vi "190717-FileSheduledROBOTPres-Ardu-TREATchoice_Prince_ArduinoWait.vi"() -> ()   [LabVIEW 2016]
uses:
  <vilib>/sound2/lvsound2.llb/Sampling Mode.ctl
  <vilib>/sound2/lvsound2.llb/Sound Data Format.ctl
  <vilib>/Utility/file.llb/Read From Spreadsheet File (string).vi
  <vilib>/Instr/_visa.llb/VISA Configure Serial Port (Instr).vi
  <vilib>/Utility/file.llb/Read From Spreadsheet File (DBL).vi
  <vilib>/sound2/lvsound2.llb/Sound Output Write (DBL).vi
panel:
  out "Numeric Control 2":i32
  out "number":i32=1
  in  "file path (dialog if empty)":path=path "C:/Users/Ralph/Documents/roboNew/RobotFiles/new files/787/RoboTutoringSchedule787.csv"
  in  "filename":string="787_undir_1766_3527_song1"
  out "all rows":string[][](array[string])=[["15:24", "787_undir_1766_3527_call1", "2", "a"], ["15:15", "787_undir_1766_3527_headmovement1", "1", "v"], ["15:16", "787_undir_1766_3527_song1", "2", "v"], ["15:17", "787_undir_1766_3527_song2", "2", "av"], ["15:18", "787_undir_1766_3527headmovement2", "3", "av"], ["15:19", "787_undir_1766_3527_call1", "4", "v"], ["15:20", "787_undir_1766_3527_song2", "2", "a"]]
  in  "Stop Button1":bool
  in  "Timer active":bool=TRUE
  in  "testPlay":bool
  in  "stop 2":bool
  out "signal":waveform(dbl)[](graph)=[{"t0"=timestamp(0 s since 1904-01-01), "dt"=0.008333333333333333, "Y"=array[729 elements]}, {"t0"=timestamp(0 s since 1904-01-01), "dt"=0.008333333333333333, "Y"=array[729 elements]}, {"t0"=timestamp(0 s since 1904-01-01), "dt"=2.0833333333333333e-05, "Y"=array[292292 elements]}, {"t0"=timestamp(0 s since 1904-01-01), "dt"=2.0833333333333333e-05, "Y"=array[292292 elements]}]
  out "Numeric 3":i32
  in  "sheduled from list":bool
  in  "play (sec)":dbl format="%#_13g"
  in  "play for (min)":dbl=30.0 format="%#_13g"
  in  "Absolute Date Time":bool=TRUE
  in  "play until":timestamp=timestamp(3577784880.043 s since 1904-01-01)
  in  "Tab Control":T1(tab)=enum."calibrations"
  in  "pause in between 1 and (sec)":dbl=6.0 format="%#_13g"
  out "Zufallszahl":dbl=1.0
  out "Numeric Control":i32=14
  in  "y":dbl=3.5
  in  "y 2":dbl=7.0
  in  "random pause":bool
  in  "constant pause":dbl=1.0
  in  "VISA resource name":refnum<visa-resource-name>="COM5"
  out "path":path=path "C:/Users/Ralph/Documents/roboNew/RobotFiles/new files/787/wav/787_undir_1766_3527_song1.wav"
  in  "excelListoutput 2":string[](array[string])
  out "Time at End":timestamp=timestamp(3646218925.390868 s since 1904-01-01)
  in  "protocol-file":path=path "C:/Users/Ralph/Documents/RobotFiles/robot1/protokol/robo1.txt"
  out "EOF? 2":bool
  in  "txt path":path=path "C:/Users/Ralph/Documents/roboNew/RobotFiles/new files/787/txt"
  in  "wav path":path=path "C:/Users/Ralph/Documents/roboNew/RobotFiles/new files/787/wav"
  in  "play clips in random order":bool=TRUE
  in  "Operation (0:Öffnen)":T2(ring)=enum."open or create"
  out "file in use 2":path=path "C:/Users/Ralph/Documents/roboNew/RobotFiles/new files/787/txt/787_undir_1766_3527_song1.txt"
  out "excelListoutput":string[](array[string])
  out "filenames":string[](array[string])=["._787_undir_1766_3527_call1.txt", "._787_undir_1766_3527_headmovement1.txt", "._787_undir_1766_3527_song1.txt", "._787_undir_1766_3527_song2.txt", "._787_undir_1766_3527headmovement2.txt", "._787_undir_1771_3532_call2.txt", "787_undir_1766_3527_call1.txt", "787_undir_1766_3527_headmovement1.txt", "787_undir_1766_3527_headmovement2.txt", "787_undir_1766_3527_song1.txt", "787_undir_1766_3527_song2.txt", "787_undir_1766_3527_song3.txt", "787_undir_1766_3527headmovement2.txt", "787_undir_1771_3532_call2.txt"]
  out "Fehler (Ausgang)":errorcluster
  out "element":i32=729
  out "size(s) 2":i32[](array[numeric])=[729, 4]
  out "Zufallszahl 2":dbl
  in  "00:00":string[](array[string])=["00:00", "902_3218_song1", "2", "2,5", "3"]
  in  "#songs if stop or manual":i32=1
  in  "delay in frames default":i32
  in  "delay in intro":i32=20
  in  "delay in frames contact":i32=35
  in  "delay in head":i32
  in  "delay in frames song":i32=19
  out "substring":string="787_un"
  in  "AttenBeak":dbl(slide)=0.5868263473053893 scale=0.0..2.0
  in  "OffsetB":dbl(slide)=4.407185628742515 scale=-2.0..8.0
  in  "AttenuateH":dbl(slide)=0.3413173652694611 scale=0.0..1.0
  in  "OffsetH":dbl(slide)=15.62874251497006 scale=0.0..30.0
  in  "Endwert Motor beak":dbl=3.0
  in  "Sampling Rate Hz":i32=120
  in  "negateBeak":bool
  in  "arduino first":bool
  in  "Endwert Motor Head":dbl
  in  "negateHead":bool=TRUE
  in  "delay movemet (samples'":dbl
  in  "wait after arduino":u32=1
  in  "wait before arduino":u32=1000
  out "error out":errorcluster
  out "error out 2":errorcluster
  out "head":dbl[](graph)=[3.25524556, 3.25294984, 3.251120901, 3.253046538, 3.254022268, 3.249303827, 3.249215039, 3.2499700590000002, 3.2493095459999997, 3.248565229, 3.2495452080000002, 3.2534044619999998, 3.256207934, 3.259231787, 3.2619914740000002, 3.264856742, 3.270676864, 3.2746376670000004, 3.284129863, 3.2956746199999998, 3.300381861, 3.312177085, 3.321709216, 3.3253852939999997, 3.327262519, 3.3293910859999998, 3.331196512, 3.331579734, 3.330605733, 3.334049257, 3.333645644, 3.334527532, 3.336280094, 3.338991439, 3.3986287020000003, 3.708982361, 4.4244339859999995, 5.395669363, 4.981378934, 5.531567489, 5.848262042, 6.068882211, 6.201616043, 6.242202127, 6.294738485, 6.294786435, 6.306837376000001, 6.284361685, 6.263991517, 6.244760256, 6.225402722, 6.220988522, 6.193365955, 6.197575853, 6.179223407, 6.186652073, 6.186890815, 6.173817251, 6.173178823, 6.175700391, 6.164617732, 6.166750807, 6.167856604, 6.167219086, 6.1790438850000005, 6.184330803, 6.183288790000001, 6.182242962, 6.199099487, 6.195969857000001, 6.201212773, 6.184360826000001, 6.194674002999999, 6.1892039510000005, 6.199708998, 6.190704289, 6.189952258, 6.18540825, 6.1763629689999995, 6.172376483000001, 6.150909639, 6.150504311, 6.14149011, 6.149450419, 6.139135842, 6.132062482, 6.132533071, 6.109822698, 6.114936618, 6.0545361589999995, 5.783199583, 6.732510575, 5.991935586, 5.328017849, 4.880723553999999, 4.649590938999999, 4.510889999, 4.42124256, 4.36307795, 4.3398573119999995, 4.3296939000000005, 4.326524216, 4.336089037, 4.352689383, 4.363369283, 4.367219745, 4.372433282, 4.384251809, 4.366195183, 4.371260579, 4.414009236, 4.412001181, 4.382009835, 4.405984394, 4.381107668, 4.3987839840000005, 4.39187896, 4.392596929, 4.387452412, 4.40148303, 4.407740435, 4.419200268, 4.418066569, 4.395799583, 4.414641294, 4.425368311, 4.4292789169999995, 4.424837557, 4.436759943, 4.427485776, 4.417763665, 4.42740788, 4.434259032, 4.443666318, 4.440932629, 4.438029218, 4.430423928, 4.437210477, 4.42934142, 4.4440042150000005, 4.46085612, 4.515481544, 4.599755559, 4.7746048, 5.147768213, 5.608406523999999, 5.970478003, 6.283057851, 6.451734065, 6.544220087999999, 6.597438406999999, 6.604634316, 6.6057426889999995, 6.607558951, 6.603214268, 6.5924813570000005, 6.585257342999999, 6.575683275, 6.567629446000001, 6.561864099, 6.554954175000001, 6.54900351, 6.540336537, 6.534894219, 6.527450622, 6.534547859, 6.533097025, 6.535607645, 6.542063542, 6.545372673, 6.545946659, 6.555789289, 6.556181849000001, 6.564339838, 6.578835991, 6.568178120000001, 6.570681201, 6.5812950699999995, 6.588320256, 6.58264089, 6.5774010050000005, 6.566674597, 6.543780782, 6.575685928, 6.549560234, 6.542357885, 6.52296925, 6.525505777, 6.48089064, 6.182235822, 5.533429566, 4.783162965, 4.176488505, 3.67093741, 3.369401742, 3.175906839, 3.058897478, 2.990157142, 2.942835441, 2.918307175, 2.9015825370000004, 2.8761458319999997, 2.862263684, 2.857263332, 2.8532595, 2.838807965, 2.844757671, 2.854599888, 2.875434345, 2.894027045, 2.9022515899999997, 2.904804833, 2.89819971, 2.906403507, 2.896207391, 2.905543123, 2.910204423, 2.919927563, 2.9279391610000003, 2.922827593, 2.918972679, 2.916615702, 2.9214819199999997, 2.910400927, 2.89788107, 2.90771033, 2.903308695, 2.90577119, 2.919475314, 2.917287667, 2.9174551209999997, 2.927137374, 2.930432183, 2.935499217, 2.929656352, 2.911943258, 2.716712348, 2.177361851, 1.6286563859999998, 2.192884673, 1.8595170579999998, 1.644114311, 1.516542643, 1.44354007, 1.387365455, 1.3916209510000002, 1.348119024, 1.34150485, 1.334830959, 1.33829409, 1.342183192, 1.374508793, 1.386269052, 1.3825264739999998, 1.381415714, 1.3999828989999998, 1.406678763, 1.400418425, 1.397494252, 1.4221112360000001, 1.430052897, 1.416414188, 1.4216419, 1.428052962, 1.4285850599999999, 1.437826446, 1.481761904, 1.486418276, 1.439962188, 1.429426635, 1.4118646570000002, 1.4207216589999998, 1.443912344, 1.431446604, 1.404633209, 1.382998974, 0.270754281, 0.269378914, 0.291119248, 0.410243505, 0.507311714, 0.43301946799999996, 0.287731185, 0.181332725, 0.095510345, 0.05501365800000001, 0.02989021, 0.017852849, 0.008676989999999999, 0.0, 0.0021227779999999996, 0.020615238, 0.029842827, 0.035963662, 0.060233327, 0.07661011399999999, 0.076688934, 0.074212782, 0.067777612, 0.07288713599999999, 0.081955573, 0.080430945, 0.087522001, 0.089051347, 0.096283761, 0.10209227, 0.10540058199999999, 0.107860207, 0.109560717, 0.11687302900000002, 0.123437048, 0.12689772900000001, 0.131027561, 0.133504854, 0.13752312, 0.152202316, 0.146481111, 0.150020031, 0.15564714899999998, 0.15567402200000002, 0.15673539, 0.158637759, 0.153910911, 0.156236087, 0.158094272, 0.163967307, 0.16597499100000002, 0.158985659, 0.124376924, 0.082897304, 0.048770680000000004, 0.106758862, 0.11858252700000001, 0.119064246, 0.11287633700000001, 0.112181202, 0.11373016899999999, 0.125524133, 0.174778548, 0.183381513, 0.186724594, 0.20124357399999998, 0.219433228, 0.259761999, 0.266871619, 0.267433663, 0.272279, 0.28117837999999995, 0.284366341, 0.28782350100000004, 0.29441447, 0.296029783, 0.30941166200000003, 0.322320873, 0.336804545, 0.3380825, 0.34098073100000004, 0.34903187900000004, 0.35024654, 0.34805977499999996, 0.320128326, 0.301662508, 0.434048818, 0.706930252, 1.175414758, 1.731252215, 2.073431367, 2.274832721, 2.359583345, 2.398444265, 2.425121622, 2.44515019, 2.467429706, 2.4701743709999997, 2.477141835, 2.470315281, 2.4509581110000003, 2.4398641540000003, 2.440090352, 2.437596091, 2.431375163, 2.431002812, 2.425480372, 2.431444036, 2.426855592, 2.422953169, 2.420014954, 2.42809091, 2.4289125489999996, 2.422944895, 2.429896007, 2.438965102, 2.425792201, 2.4219395340000003, 2.424806909, 2.4306000809999997, 2.419801867, 2.42394656, 2.4458672839999998, 2.44346788, 2.4774497930000003, 2.505235061, 2.513905079, 2.505880531, 2.522745288, 2.5670542239999996, 2.57367299, 2.576946799, 2.585496921, 2.640307362, 2.88926106, 3.3845219309999997, 4.022265457, 4.441104297, 4.7763219, 4.940020379, 5.029538535, 5.07945522, 5.089948507, 5.097297681000001, 5.087985588, 5.079381132, 5.073041596, 5.056952103, 5.0441750800000005, 5.032143137, 5.016805661, 5.027118635, 5.021018191, 5.015767505, 5.004121598, 4.997389138, 4.999753569999999, 5.003682355, 5.001514196, 4.989545148, 5.013715413, 5.022027724, 5.011709822, 5.022139255, 5.014835049, 5.027755824, 5.024893426, 5.010810833000001, 4.997868701, 5.005595357, 5.006128596, 5.006788031, 5.004479172, 5.003432070000001, 5.008701481, 5.010254025, 5.013583799, 5.014878442, 5.012146706, 5.019084469, 4.955066683, 4.753923657, 4.1712075440000005, 3.5681203320000003, 3.0596109460000003, 2.611292663, 2.327130841, 2.149094549, 2.063565686, 2.005586268, 1.975166431, 1.9870035080000001, 1.986147625, 1.980409529, 1.9965147719999998, 1.9954128320000002, 1.9942562009999998, 1.997415518, 2.001347313, 2.004257857, 2.0157028429999997, 2.004202592, 1.995414309, 2.001979945, 1.9901548379999998, 1.964929078, 1.965143012, 1.9928702010000001, 1.992531296, 1.984086013, 1.995151802, 2.0044798480000003, 2.0027663880000004, 1.9981825359999998, 2.015886754, 1.989362942, 1.984461507, 1.9924783689999999, 1.974517622, 1.9876329410000002, 1.986738481, 1.9990147729999999, 1.997448033, 1.965123251, 1.932786674, 1.826887741, 1.464959993, 0.9771017830000001, 1.499997478, 1.0315501, 0.7725876269999999, 0.552059249, 0.404394452, 0.3123435, 0.265544699, 0.259630798, 0.25745608, 0.29851654699999997, 0.298042318, 0.308826413, 0.292164985, 0.303818102, 0.293371813, 0.318218187, 0.306813962, 0.310613856, 0.29662472, 0.29811298999999997, 0.28947382099999996, 0.263475009, 0.263837679, 0.259598024, 0.250143537, 0.278838077, 0.284727562, 0.281413419, 0.265428534, 0.244827513, 0.24707295199999998, 0.26250665, 0.257333104, 0.26590648, 0.369826618, 0.765838724, 0.001103501, 0.40339962599999996, 0.84245658, 1.0872724589999998, 1.247521464, 1.361242281, 1.4383747, 1.486031701, 1.50842174, 1.522843084, 1.4653872030000001, 1.515033758, 1.499154083, 1.46092247, 1.493913253, 1.454899922, 1.453957372, 1.483851159, 1.488892916, 1.501597797, 1.493513217, 1.481620063, 1.4837993310000002, 1.483951553, 1.477027888, 1.5231720210000002, 1.51360097, 1.5118852839999999, 1.486021747, 1.492590582, 1.489181638, 1.505135723, 1.4983500209999998, 1.49058945, 1.498207788, 1.493478553, 1.506093988, 1.50738812, 1.501032379, 1.488595787, 1.470975184, 1.485354283, 1.488374377, 1.507590462, 1.531567779, 1.5214578680000002, 1.539273141, 1.703207247, 2.288336995, 3.3042687159999997, 4.496766673, 5.364422931, 6.054205906, 6.453892088, 6.717023845, 6.852505107, 6.92372037, 6.971750261, 7.0, 6.998607000000001, 6.996479322, 6.985190961, 6.96481695, 6.941319224, 6.927206335, 6.908007141, 6.887833659, 6.874964019, 6.875516711, 6.8688117890000004, 6.864254502, 6.860387772, 6.858015234, 6.850694732, 6.85145678, 6.847559089, 6.841938537, 6.836315717, 6.8383274400000005, 6.8322527, 6.830337332, 6.817685763, 6.809278399, 6.801957273999999, 6.797368767, 6.806043321, 6.790130872, 6.7905920879999995, 6.786451826, 6.782634054, 6.780588563, 6.7752516510000005, 6.772797682, 6.773018273, 6.773639278, 6.77358878, 6.768301617, 6.763453802, 6.767610962, 6.771605267, 6.766666445, 6.76777297, 6.771644964, 6.769827414, 6.770487157, 6.759561291, 6.7571161769999994, 6.758021186, 6.751027465, 6.748728973, 6.7525185489999995, 6.738689461, 6.7379110749999995, 6.732918457999999, 6.726450906, 6.6280645410000005, 6.174074074, 5.53941045, 5.0944223609999995, 4.967646537, 5.651245599999999, 5.6314190239999995, 5.640855017, 5.648209371, 5.652477964, 5.652267782, 5.652233734, 5.651315544, 5.654595128, 5.65505451, 5.65888407, 5.658570064, 5.658802226, 5.6578705959999995, 5.658150435, 5.655382922, 5.653845582, 5.650123269, 5.649389445, 5.648242131, 5.65034694, 5.649739921, 5.651674798, 5.649980945, 5.648781319999999, 5.647930834, 5.6385875279999995, 5.617268153, 5.606072437, 5.600720216, 5.602347324, 5.590922861999999, 5.574235275, 5.574414545, 5.5694468409999995, 5.571631506, 5.574122645, 5.576012078, 5.574806636, 5.574329789, 5.576530673, 5.573952097, 5.571414009, 5.568913308, 5.568346398999999, 5.566258047, 5.564306741, 5.560788555, 5.5583995250000005, 5.562696902, 5.563827395000001, 5.572272076, 5.646733386, 5.655266484, 5.795391406, 5.953758776, 6.118533876000001, 6.160290367, 6.174670418000001, 6.303698254, 6.192560157, 6.149822049, 6.171945255000001, 6.178014094, 6.306209826, 6.291947396, 6.298646907, 6.291803531999999, 6.327769084]
  out "head 2":dbl[](graph)=[6.0914441198823415, 6.098170176724448, 6.1035286471279555, 6.097886868549008, 6.095028150829711, 6.1088523551630445, 6.1091124884262005, 6.1069004122858495, 6.108835599496377, 6.111016317724447, 6.108145151180587, 6.096838214022693, 6.088624532899885, 6.0797651741104115, 6.071679775356026, 6.063285042794622, 6.046233106408657, 6.034628648496376, 6.006818179513921, 5.972994066899886, 5.95920267660164, 5.924644739619184, 5.896717268092868, 5.885947004478833, 5.880447064566551, 5.87421073668936, 5.868921155250764, 5.867798382022693, 5.870652034075324, 5.860563112882341, 5.8617456281630425, 5.859161851040236, 5.854027151847253, 5.846083386671815, 5.671356668759534, 4.762074895899886, 2.665927152478835, -0.17962210995976235, 1.0341761644788328, -0.577779777363272, -1.5056392572053774, -2.1520176470825696, -2.540904488205374, -2.659814593959762, -2.813736905994851, -2.8138773910825705, -2.849184534012398, -2.78333470248608, -2.723653683959764, -2.667309463135201, -2.6105952845737974, -2.59766245299485, -2.516733177749238, -2.529067440310641, -2.4752979932580104, -2.4970626813632713, -2.4977621535387087, -2.4594589046264304, -2.4575884225913427, -2.4649761744509924, -2.4325059279071297, -2.438755463433445, -2.441995254643974, -2.4401274387492364, -2.474772025293099, -2.490261767503622, -2.487208852222924, -2.4841447596615183, -2.533531420626428, -2.5243621537843275, -2.539722977854499, -2.4903497296264305, -2.520565528907131, -2.504539236205378, -2.5353171809246753, -2.5089349633281834, -2.5067316444334473, -2.4934184981878325, -2.466917411749236, -2.4552377071527474, -2.392343620345727, -2.3911560804159038, -2.3647460529246764, -2.3880683617492373, -2.3578484607141483, -2.3371247568545, -2.338503500065027, -2.2719660914509916, -2.2869489798720437, -2.109986231573796, -1.315017666801868, -4.096332327573798, -1.9265775352404653, 0.018584957373569466, 1.3290787690402386, 2.006256781408659, 2.4126262021104132, 2.6752774707595357, 2.845689573741991, 2.9137219692858523, 2.9434989833911125, 2.9527856014262017, 2.924762353934973, 2.876126252496375, 2.8448360191630435, 2.8335548410226927, 2.8182800922683064, 2.7836538815840957, 2.836556627934973, 2.8217159063209376, 2.6964698410753236, 2.7023530899349737, 2.7902224720753246, 2.7199812202683074, 2.792865663110412, 2.7410771583384808, 2.7613076672507635, 2.759204144040238, 2.774276676303394, 2.7331694270753246, 2.714836328215675, 2.6812610280226927, 2.6845825671981327, 2.74982092968936, 2.694618022022693, 2.6631897441455, 2.6517323546367297, 2.6647447602507626, 2.6298142609174295, 2.6569859431805867, 2.6854700227770785, 2.657214164794624, 2.637141491391114, 2.6095797938121663, 2.6175890229876053, 2.626095507847255, 2.648377673285852, 2.6284942753384826, 2.651549231812167, 2.6085898148823397, 2.559216689706904, 2.399173780794623, 2.152265701759534, 1.6399881009349748, 0.5466847681104117, -0.8029046693808155, -1.8637105815387116, -2.779514697608885, -3.2737064123106414, -3.544674234082567, -3.7005945722053752, -3.7216773231352036, -3.724924661573798, -3.7302459905913423, -3.7175168316264298, -3.6860712853632727, -3.6649061917141488, -3.636855852135202, -3.6132595461176606, -3.596368090872044, -3.5761232258194156, -3.5586888213457293, -3.5332961109773073, -3.517351074029939, -3.4955426407141488, -3.516336299994851, -3.512085610907132, -3.5194412870474814, -3.5383559326439737, -3.5480511059246744, -3.5497327842053785, -3.5785699633281816, -3.5797200952580113, -3.6036215718018703, -3.64609275690713, -3.614867064679064, -3.6222006528720456, -3.6532974269597602, -3.6738799894509917, -3.6572404434509913, -3.6418884996790624, -3.610462006065024, -3.5433871445737957, -3.6368636249597657, -3.5603199249948503, -3.5392183059948508, -3.4824130069597636, -3.4898445860650256, -3.359130061872044, -2.4841238407141475, -0.5832353362930967, 1.6149141789174308, 3.39236391260164, 4.873539927777079, 5.756986534022692, 6.323892653338483, 6.666709553110412, 6.868106677882341, 7.006750959759534, 7.078614475934973, 7.127614731127954, 7.202139814198132, 7.242812072373569, 7.257462226478832, 7.269192751812167, 7.3115332140051486, 7.294101619233219, 7.265265650127956, 7.20422434628585, 7.149750997163043, 7.125654523215676, 7.118173969163044, 7.137525820759535, 7.113490134812167, 7.143362965899886, 7.1160109089876045, 7.102354117759534, 7.07386702337357, 7.050394446777078, 7.065370444250762, 7.0766646659700605, 7.083570195075325, 7.069313030057781, 7.1017783955139215, 7.13845938005778, 7.109661372689359, 7.122557391022692, 7.11534271268936, 7.07519203360164, 7.081601455513921, 7.081110844671816, 7.052743542022693, 7.043090329689358, 7.028244809022693, 7.045363378408657, 7.097259636268307, 7.669251951531464, 9.249454284847253, 10.857065033180588, 9.203975139689359, 10.18068376609287, 10.811776024847253, 11.185538631092868, 11.39942336251392, 11.564005129268306, 11.551537272566552, 11.678990286759534, 11.69836865619813, 11.71792198597006, 11.707775619706903, 11.696381233145498, 11.60167289337357, 11.567217397706901, 11.578182494654271, 11.581436826584095, 11.527038231934974, 11.507420525127955, 11.525762217163043, 11.534329531040235, 11.46220608668936, 11.438938413233219, 11.478897437847253, 11.46358115882971, 11.44479787191743, 11.443238918127957, 11.416163278443744, 11.287440094478832, 11.2737977414262, 11.409905929075324, 11.440773251022692, 11.49222676551392, 11.46627730351392, 11.39833266500515, 11.434855096233218, 11.513413639478832, 11.576798152549008, 14.835479972391113, 14.839509556408657, 14.775814191882342, 14.426801017864797, 14.142408195005148, 14.36007144205778, 14.785740622075323, 15.097469443478833, 15.348913960320937, 15.467562148549007, 15.541169443566552, 15.576436799478833, 15.603320456549008, 15.62874251497006, 15.622523147847254, 15.568343484338481, 15.541308267443744, 15.523375294724445, 15.452269434110411, 15.404288321320937, 15.404057392549008, 15.411312083496377, 15.430166002619183, 15.415195993706902, 15.388627064250763, 15.393093956812166, 15.372318406777078, 15.367837691303393, 15.346647987127955, 15.329630074794622, 15.319937301040236, 15.312731031303393, 15.307748835338481, 15.286325044040236, 15.267093619952517, 15.256954431759533, 15.244854748531464, 15.237596714654272, 15.225823900233218, 15.182816431250762, 15.199578558180587, 15.189210143443745, 15.172723674917428, 15.17264494174199, 15.169535319706902, 15.16396171228585, 15.177810547654271, 15.170998189899885, 15.165554033847254, 15.148347071654271, 15.142464909759534, 15.162942426320937, 15.264339948163043, 15.385867957636727, 15.48585297882971, 15.315957778934973, 15.281316514812165, 15.279905162654272, 15.298034650426201, 15.300071274022692, 15.29553307246129, 15.26097882705778, 15.116672032233218, 15.091466854075323, 15.081672213250762, 15.039134149040235, 14.985841653987604, 14.867685430180586, 14.84685549088234, 14.845208800566551, 14.831012813215674, 14.804939191110412, 14.795599024671814, 14.785470152391113, 14.766159769531464, 14.76142718582971, 14.72222062805778, 14.68439890460164, 14.641964286636727, 14.638220102689358, 14.629728794320938, 14.606140343163043, 14.602581599531463, 14.608988437338482, 14.690822682654272, 14.744924289777078, 14.357055627145499, 13.557560899461288, 12.184983487145498, 10.556477253478832, 9.553952369549009, 8.963881735899886, 8.715577276110412, 8.601721598215676, 8.523561622443745, 8.464881431987603, 8.399606358794623, 8.391564971864799, 8.371151524706903, 8.39115213028585, 8.447865242391114, 8.480368590092866, 8.479705869636728, 8.487013616777078, 8.505239844426201, 8.506330767531464, 8.52251054788234, 8.505038058619185, 8.518481394549008, 8.529914809303396, 8.538523263777078, 8.514862129531465, 8.512454871408657, 8.529939050671814, 8.509573512005149, 8.483002654724448, 8.521596943619183, 8.532884582022692, 8.524483676320937, 8.507510698706904, 8.539147571303396, 8.527004347952516, 8.46278047237357, 8.469810305145499, 8.370249261794621, 8.288843301163043, 8.263441669478834, 8.286952187303395, 8.237541408022693, 8.107723999040237, 8.088332175847254, 8.078740489829709, 8.053690132391115, 7.893105156127955, 7.163714497075324, 5.712687032917431, 3.8442103865665533, 2.6170860658647985, 1.6349572991805879, 1.1553494747419908, 0.8930769826016398, 0.7468298528647992, 0.7160863628823417, 0.6945545723911124, 0.7218373711805892, 0.7470469177069035, 0.7656206459876049, 0.8127600377595332, 0.8501944735665514, 0.8854459556893595, 0.9303820695840965, 0.9001668650577805, 0.9180400957244483, 0.9334236845314638, 0.9675441488998846, 0.9872690755665534, 0.9803417046191854, 0.968831053829712, 0.9751833793209403, 1.0102505901279546, 0.939435954075325, 0.9150823411454994, 0.9453119838472528, 0.9147555748823422, 0.9361556170226919, 0.8983000130753247, 0.9066863370402363, 0.9479458638998839, 0.9858640401104122, 0.9632262935840963, 0.9616639968647984, 0.9597319680051495, 0.9664965198121678, 0.9695643449700597, 0.954125895198132, 0.9495772136542726, 0.9398215600051483, 0.9360284831455008, 0.9440319903735688, 0.9237055619349732, 1.111266443724448, 1.7005802216542723, 3.407836201847253, 5.174775928233219, 6.664619217040235, 7.978113133899885, 8.810657419408658, 9.332272520531465, 9.58285708405778, 9.75272660697006, 9.841851392566552, 9.807170833636727, 9.809678420671816, 9.826490035268307, 9.779304498759535, 9.782532989636728, 9.785921715549009, 9.776665471005149, 9.765146001443744, 9.756618618145499, 9.72308681705778, 9.756780534899885, 9.78252866228585, 9.763292500671815, 9.797937989601639, 9.87184504082971, 9.87121825174199, 9.789982452391113, 9.790975384584097, 9.8157185821455, 9.783297761741991, 9.755968223461288, 9.76098836065427, 9.77441824282971, 9.722547990092869, 9.800258105952516, 9.814618450601639, 9.791130451408659, 9.843752289110412, 9.80532670537357, 9.807947316250763, 9.771979934426202, 9.776570207759534, 9.871276148005148, 9.966016645531464, 10.276281940461288, 11.336666746005148, 12.7660057121455, 11.23401306188234, 12.606481695671814, 13.365196309549008, 14.011305767899884, 14.443937717005149, 14.713630857075323, 14.850743133689358, 14.868069826092867, 14.874441368303394, 14.754141403584095, 14.755530811356024, 14.723935304952516, 14.772750365934973, 14.738608777531464, 14.769214571619184, 14.696419054812166, 14.729831433320937, 14.718698410549008, 14.75968412479462, 14.755323754794622, 14.780635004320938, 14.85680696228585, 14.855744402812165, 14.868165848163043, 14.895865836391113, 14.811795868320937, 14.79454071051392, 14.804250568075323, 14.851083476759534, 14.911440854075323, 14.90486211174199, 14.859644084268306, 14.874801666408658, 14.849683178829709, 14.545215406092867, 13.384969411320938, 15.625509450636727, 14.44685238265427, 13.16049253497006, 12.443224959654271, 11.973723488864797, 11.640541446075323, 11.414556990408657, 11.274930338356025, 11.209331452163044, 11.167079444303393, 11.33541509565427, 11.1899593994262, 11.236484061268307, 11.34849598005778, 11.251838773724447, 11.366140989110411, 11.368902495250762, 11.281318943864797, 11.26654748037357, 11.229324407970061, 11.253010809022692, 11.287855663724446, 11.281470790812165, 11.28102480705778, 11.30130993082971, 11.166115716601638, 11.194157216899885, 11.19918387588234, 11.27495950182971, 11.255713967706903, 11.265701575566553, 11.218958905478832, 11.238839821864797, 11.261576933391112, 11.23925653960164, 11.253112368461288, 11.216151357145499, 11.212359777426201, 11.23098098351392, 11.267418016215675, 11.319043291671814, 11.276915054250763, 11.268066708671814, 11.211766950864797, 11.14151761860164, 11.171137884163041, 11.118942259759535, 10.638644089549008, 8.924316582250764, 5.947814873356027, 2.454005069513922, -0.08807554602993939, -2.1090186482229214, -3.2800290411001143, -4.050958925643972, -4.447895254661518, -4.656543481345729, -4.797262635679061, -4.880029414854498, -4.875948169240466, -4.869714445977305, -4.8366415286615165, -4.776949250819413, -4.708105036047481, -4.666756747222919, -4.61050647708257, -4.551401714029939, -4.513695926661516, -4.51531521725801, -4.495670972100115, -4.482318920714146, -4.470990080187832, -4.4640389600825685, -4.442591173521166, -4.444823840468537, -4.433404289643974, -4.416937058345727, -4.400463182205375, -4.406357177661519, -4.388559255205376, -4.38294756299485, -4.34588068539836, -4.321248583854501, -4.299798972012393, -4.286355451503624, -4.311770372872044, -4.265149688959763, -4.266500970924675, -4.25437072962643, -4.243185327450991, -4.237192397679063, -4.2215561818194125, -4.214366483170291, -4.215012776100114, -4.216832211801869, -4.216684261521166, -4.201193801503621, -4.186990554047483, -4.199170303521168, -4.210872916415902, -4.196403034415905, -4.199644958538713, -4.210989221661517, -4.205664119029937, -4.207597050275552, -4.1755861797141485, -4.1684224246615145, -4.171073942258008, -4.1505835666966036, -4.143849388380815, -4.154952181222921, -4.114435379538708, -4.112154845117654, -4.0975273532053755, -4.078578560503622, -3.7903237718194127, -2.4602113509597636, -0.6007582771352027, 0.7029787555490099, 1.0744096784963766, -0.9284156464334465, -0.8703272571001115, -0.8979730611527437, -0.919520028135203, -0.9320262567492357, -0.9314104603632707, -0.9313107056966068, -0.9286205700825718, -0.938229175836959, -0.9395750845036233, -0.9507950234509899, -0.949875040959764, -0.9505552348895883, -0.9478257224334463, -0.9486456016088844, -0.9405372740474824, -0.9360331375562545, -0.9251274135036205, -0.9229774379246756, -0.919616009187834, -0.925782730293097, -0.9240042711176564, -0.9296731212755525, -0.9247104291527464, -0.9211957383632701, -0.9187039635913443, -0.8913297161878333, -0.828867687679061, -0.7960662039597644, -0.780385135415905, -0.7851522763983603, -0.751680607029936, -0.7027889047667806, -0.7033141344159013, -0.6887596332229187, -0.6951603183983615, -0.7024589186264301, -0.7079946258369567, -0.7044628922580074, -0.7030658142053774, -0.7095140182053754, -0.7019592429071331, -0.6945230903457258, -0.6871964751352024, -0.6855355312229179, -0.6794170262404648, -0.6737000419948522, -0.6633923742404662, -0.6563929354685349, -0.6689834961527446, -0.6722956423106403, -0.6970370761176561, -0.9151956510299399, -0.9401961311352025, -1.3507375692755517, -1.8147261796264296, -2.297488314714151, -2.419827507643973, -2.4619585342580095, -2.839987457275555, -2.514372330977306, -2.3891571724509895, -2.453974284766783, -2.471754918328184, -2.847345922608884, -2.8055595048895867, -2.8251878967667814, -2.8051380086088855, -2.91051076622292]
  out "beak 2":dbl[](graph)=[1.5571000855431985, 1.5571000855431985, 1.5571000855431985, 1.5571000855431985, 1.5571000855431985, 1.5571000855431985, 1.5571000855431985, 1.5571000855431985, 1.5571000855431985, 1.5571000855431985, 1.5571000855431985, 1.5571000855431985, 1.5571000855431985, 1.5571000855431985, 1.5571000855431985, 1.5571000855431985, 1.5571000855431985, 1.5571000855431985, 1.5571000855431985, 1.5571000855431985, 1.5571000855431985, 1.5571000855431985, 1.5571000855431985, 1.5571000855431985, 1.5571000855431985, 1.5571000855431985, 1.5571000855431985, 1.5571000855431985, 1.5571000855431985, 1.5571000855431985, 1.5571000855431985, 1.5571000855431985, 1.5571000855431985, 1.5571000855431985, 1.5571000855431985, 1.5571000855431985, 1.5571000855431985, 1.5571000855431985, 1.5571000855431985, 1.5571000855431985, 1.5571000855431985, 1.5571000855431985, 1.5571000855431985, 1.5571000855431985, 1.5571000855431985, 1.5571000855431985, 1.5571000855431985, 1.5571000855431985, 1.5571000855431985, 1.5571000855431985, 1.5571000855431985, 1.5571000855431985, 1.5571000855431985, 1.5571000855431985, 1.5571000855431985, 1.5571000855431985, 1.5571000855431985, 1.5571000855431985, 1.5571000855431985, 1.5571000855431985, 1.5571000855431985, 1.5571000855431985, 1.5571000855431985, 1.5571000855431985, 1.5571000855431985, 1.5571000855431985, 1.5571000855431985, 1.5571000855431985, 1.5571000855431985, 1.5571000855431985, 1.5571000855431985, 1.5571000855431985, 1.5571000855431985, 1.5571000855431985, 1.5571000855431985, 1.5571000855431985, 1.5571000855431985, 1.5571000855431985, 1.5571000855431985, 1.5571000855431985, 1.5571000855431985, 1.5571000855431985, 1.5571000855431985, 1.5571000855431985, 1.5571000855431985, 1.5571000855431985, 1.5571000855431985, 1.5571000855431985, 1.5571000855431985, 1.5571000855431985, 1.5571000855431985, 1.5571000855431985, 1.5571000855431985, 1.5571000855431985, 1.5571000855431985, 1.5571000855431985, 1.5571000855431985, 1.5571000855431985, 1.5571000855431985, 1.5571000855431985, 1.5571000855431985, -1.0355676439925157, -1.0157922375996584, -0.9551481796710872, -1.0312321569925156, -1.0883134905996585, -1.1538406464210866, -1.3794717996710872, -1.4992542793139436, -1.9474588098496581, -1.9666742771710863, -2.1589275102068006, -2.483124759313944, -2.1437719739210865, -1.9862232315639439, -1.7444240627782297, -1.8747330892068006, -2.9958904997782296, -3.098860498956801, -2.9911354014210865, -4.093932253456801, -4.045241059492515, -4.037915067706801, -3.6791704272068007, -3.260240030456801, -2.900140292313943, -2.6117954739925153, -2.5003050811353726, -3.9354332035639437, -3.1894905818496584, -2.899313874921086, -3.5878858832425156, -3.0730358336710863, -2.868620640742515, -2.6946449553139438, -2.4429381536710864, -1.997079841921087, -2.142226365063944, -2.3685166017068013, -2.784649336921087, -2.1229865157425154, -1.9168238169210867, -2.999887692492515, -3.2873835722782294, -3.0548865480282297, -3.015418370421087, -3.0724014483853725, -3.412357324456801, -3.5267763724568004, -3.744059654956801, -3.518400648492515, -3.518400648492515, -3.518400648492515, -3.518400648492515, -3.518400648492515, -2.7727462628139437, -2.9854852128853726, -3.247799687528229, -2.8302742558139444, -2.266827438849658, -2.3383878990996587, -3.7321482487425155, -4.329985638135372, -4.398364545599658, -3.533035943992515, -3.317767325635373, -4.118459465921086, -4.2684815719568014, -4.1775044332425155, -3.353294368849658, -3.205433338242515, -3.1947066061710867, -3.0887172589210863, -2.820415595706801, -2.625221677563944, -2.69831211427823, -3.2139827243139436, -3.1916167840996583, -2.386169986813944, -2.717376756742515, -4.407185628742515, -4.0713135050639435, -3.7875534570282294, -3.2593991794925152, -2.535819324992515, -2.0072149466710867, -2.189211087421086, -2.259882791563944, -2.389590671671087, -3.4783090539210866, -3.518400648492515, -1.826567068492515, -0.1347334944568015, 0.711183295543198, 0.711183295543198, 0.711183295543198, 0.711183295543198, 0.711183295543198, -0.07842613427823064, -0.3956979470639439, -0.6320136231353723, -0.9605526455996585, -1.024075336206801, -0.9732782125996589, -1.1282546658853727, -1.4973572726353725, -1.2239411509210867, -1.1310137027068015, -1.1106717309210867, -1.0393858663853726, -0.5796655526353729, -0.05796171570680109, 0.18272165450748368, -0.6992666225639446, -1.315297624171087, -0.620931920635373, -1.7166333422782296, -2.308091790921087, -2.039171905635372, -1.759189147099658, -1.4209821308139436, -1.0421738061353727, -0.8893002347425156, -0.7040949921710871, -1.62825635777823, -1.694048214563944, -1.2420645575282294, -1.674336620063944, -1.6162842112782294, -1.4473275140282298, -1.4422686963496583, -1.0630196467425153, -0.5685295989925154, -0.41333836581394445, -0.7118816295996591, -0.4177122329925158, -0.23867078745680192, 0.711183295543198, 0.711183295543198, 0.711183295543198, 0.711183295543198, 0.711183295543198, -0.1187802468853727, -0.16561076263537267, -0.5820992734568011, -0.64794297777823, -0.457604948456801, -0.27566821199251557, -0.2597423404925161, -0.18761624527822995, -0.0755585892068007, -0.032040780885372655, 0.19921038757891285, -0.6702745756353727, -0.9021103633853729, 0.1297480914717708, 1.3555630302574837, 0.36648090372176956, -1.5291586651353728, -2.3814538590996586, -3.0652222853853726, -1.0353523929210873, -0.788470131813944, -2.0013345128496582, -2.3257003305639437, -2.06396340752823, -1.7162915469568008, -1.2267893597782296, -0.7466774275282302, -0.2907077130996587, -0.17585384481394417, -0.10243141806394451, -0.21285112620680113, -0.42924444781394433, -0.6119521397782295, -0.06485233849251504, 0.7909401992931988, -1.656327632313944, -3.145714973242515, -3.2386397375282296, -1.2023785642068012, 0.3275425276503414, 1.5571000855431985, 1.5571000855431985, 1.5571000855431985, 1.5571000855431985, 1.5571000855431985, 1.5571000855431985, 1.5571000855431985, 1.5571000855431985, 1.5571000855431985, 1.5571000855431985, 1.5571000855431985, 1.5571000855431985, 1.5571000855431985, 1.5571000855431985, 1.5571000855431985, 1.5571000855431985, 1.5571000855431985, 1.5571000855431985, 1.5571000855431985, 1.5571000855431985, 1.5571000855431985, 1.5571000855431985, 1.5571000855431985, 1.5571000855431985, 1.5571000855431985, 1.5571000855431985, 1.5571000855431985, 1.5571000855431985, 1.5571000855431985, 1.5571000855431985, 1.5571000855431985, 1.5571000855431985, 1.5571000855431985, 1.5571000855431985, 1.5571000855431985, 1.5571000855431985, 1.5571000855431985, 1.5571000855431985, 1.5571000855431985, 1.5571000855431985, 1.5571000855431985, 1.5571000855431985, 1.5571000855431985, 1.5571000855431985, 1.5571000855431985, 1.5571000855431985, 1.5571000855431985, 1.5571000855431985, 1.5571000855431985, 1.5571000855431985, 1.5571000855431985, 1.5571000855431985, 1.5571000855431985, 1.5571000855431985, 1.5571000855431985, 1.5571000855431985, 1.5571000855431985, 1.5571000855431985, 1.5571000855431985, 1.5571000855431985, 1.5571000855431985, 1.5571000855431985, 1.5571000855431985, 1.5571000855431985, 1.5571000855431985, 1.5571000855431985, 1.5571000855431985, 1.5571000855431985, 1.5571000855431985, 1.5571000855431985, 1.5571000855431985, 1.5571000855431985, 1.5571000855431985, 1.5571000855431985, 1.5571000855431985, 1.5571000855431985, 1.5571000855431985, 1.5571000855431985, 1.5571000855431985, 1.5571000855431985, 1.5571000855431985, 1.5571000855431985, 1.5571000855431985, 1.5571000855431985, 1.5571000855431985, 1.5571000855431985, 1.5571000855431985, 1.5571000855431985, 1.5571000855431985, 1.5571000855431985, 1.5571000855431985, 1.5571000855431985, 1.5571000855431985, 1.5571000855431985, 1.5571000855431985, 1.5571000855431985, 1.5571000855431985, 1.5571000855431985, 1.5571000855431985, 1.5571000855431985, 1.5571000855431985, 1.5571000855431985, 1.5571000855431985, 1.5571000855431985, 1.5571000855431985, 1.1300264228646268, 0.6788234431146272, 0.7742923510074844, 0.45386793607891285, 0.21371152840034124, 0.534501393007484, 0.9197063783289128, 1.1027557463289126, 0.9977657330431988, -0.07316940370680136, -0.05617172620680133, -0.004595541635372236, -1.3581847331353725, -1.515719721849658, -0.8112765225996585, -0.6040285921710868, -0.38386745831394453, -0.18581073670680137, 0.15720398890034115, 0.09183714115034203, -0.9545712125639438, -0.40604811202823043, -0.20557889052822986, -0.6986478517782295, -0.05390456402822963, 0.14655462554319865, -0.22258343292108673, 0.24142484440034107, 0.7934047017931984, 0.4728811842931986, 0.26312856997177025, 0.25465873554319796, 0.7519358164717707, 1.0443829301503413, 0.11498920404319879, -0.015148575813944909, 0.0794564231860555, 0.13885036086462677, 0.19317870543605586, 0.09230858811462728, -0.0771101205996585, -0.09861117377823003, 0.04560252315034141, 0.16806599097176989, 0.19900058786462704, 0.5156491685789133, 0.5506988005431985, 0.47063696075748496, 0.19290131843605618, -0.17706279956394422, 0.5803832175431989, 1.2790385307931986, 1.5571000855431985, -0.12349782988537239, -1.1375598283496582, -1.6947796805282302, -0.72074266152823, -0.4165059860282301, -0.5517814373853729, -1.2363427677425158, -1.165620218063944, -0.4199097144210868, -0.17766166752822965, -0.030463149778229948, 0.5752027165074844, 0.5913740422217701, 0.29918050015034137, 0.27363042461462683, 0.19569269957891322, 0.5415170033646266, 1.5239406669360553, -3.180033932492515, -3.518400648492515, -2.5511063976353725, -1.8733555419925154, -1.2195475479210867, -0.3605233990996579, 0.08377263957891312, 0.5088425467931978, 0.025530811043198653, -0.46364600049251514, -1.4942951785282297, -1.6898488504568014, -1.0946882265282296, -1.5112848817782294, -1.4950442808853723, -1.0549204747782297, -0.6854752138496591, -0.6038763597425159, -0.2584471123496579, -0.04291369759965846, -0.08693985988537278, -0.18358936831394423, -0.550361000992516, -0.8692802270282294, -1.093740728171087, -1.2606022135996584, -1.206184541921087, -1.72034141027823, -1.4363718368853724, -1.4518724667425156, -1.4851852748496581, -1.0675156863496582, -0.502555938849659, -0.030385184635372653, -0.11499590163537299, -1.5007353128496583, -1.6856679219568016, -1.3042314884568014, -2.621248163063944, -2.5297169600996585, -2.500472170599658, -2.0765660804210864, -1.5311282869925154, -1.4970804403139444, -2.672483858492516, -4.364317438492515, -2.672483858492516, -3.003767293349658, -1.8889071008853722, -2.0800523485639437, -2.148561539885373, -1.9550356535282294, -2.065977033885373, -1.935244006385373, -1.0252442407782296, -1.16541535677823, -1.7023998845639445, -0.9058590541353726, -1.0956438482425157, -0.14396267192108692, -0.9212214676353727, -1.248563958956801, -2.040073956135373, -1.532209110992515, -1.2490318989210873, -1.1787785297782296, -1.3682679187782294, -1.7171406167068013, -1.849730904885372, -2.4478391444210867, -1.6870876187782295, -1.6137660838853725, -1.599581264921087, -1.5129997153139443, -1.6002154414568008, -2.0999369312068006, -2.5540910156710863, -1.6425331102425154, -0.9939769858496588, -0.8694804063496586, -2.393090240171087, -2.870706238135373, -4.364317438492515, -2.672483858492516, -1.488200358456801, -1.826567068492515, -3.180033932492515, -2.9787122654568012, -2.5065643723496582, -2.176055948706801, -2.0700205094568016, -1.915859910813944, -1.7070287607425159, -1.822108949813944, -1.93840717127823, -2.001623243921087, -2.028552805063944, -1.978700913385373, -2.232619331813944, -3.1878910856710867, -4.276552097456801, -4.250343988242515, -3.493212372492515, -2.474407872242516, -1.5788735452425153, -1.2248667842068013, -1.4318253215282297, -1.3475401769925153, -1.2639447543853728, -2.0043904279568006, -2.8105974211710865, -2.264156303671087, -2.8109793322782295, -2.8810995308496583, -1.998171848956801, -1.9289641264568016, -1.9815591720639438, -1.532637436171087, -1.089398936921087, -1.1134762812068013, -1.3822605445996583, -1.6970397511710873, -1.6048733159925157, -1.8342147857782294, -1.6302087488139438, -1.3189444031710869, -1.4873568295282302, -1.2687753904210872, 1.5571000855431985, 1.5571000855431985, 1.5571000855431985, 1.5571000855431985, 1.5571000855431985, 1.5571000855431985, 1.5571000855431985, 1.5571000855431985, 1.5571000855431985, 1.5571000855431985, 1.5571000855431985, 1.5571000855431985, 1.5571000855431985, 1.5571000855431985, 1.5571000855431985, 1.5571000855431985, 1.5571000855431985, 1.5571000855431985, 1.5571000855431985, 1.5571000855431985, 1.5571000855431985, 1.5571000855431985, 1.5571000855431985, 1.5571000855431985, 1.5571000855431985, 1.5571000855431985, 1.5571000855431985, 1.5571000855431985, 1.5571000855431985, 1.5571000855431985, 1.5571000855431985, 1.5571000855431985, 1.5571000855431985, 1.5571000855431985, 1.5571000855431985, 1.5571000855431985, 1.5571000855431985, 1.5571000855431985, 1.5571000855431985, 1.5571000855431985, 1.5571000855431985, 1.5571000855431985, 1.5571000855431985, 1.5571000855431985, 1.5571000855431985, 1.5571000855431985, 1.5571000855431985, 1.5571000855431985, 1.5571000855431985, 1.5571000855431985, 1.5571000855431985, 1.5571000855431985, 1.5571000855431985, 1.5571000855431985, 1.5571000855431985, 1.5571000855431985, 1.5571000855431985, 1.5571000855431985, 1.5571000855431985, 1.5571000855431985, 1.5571000855431985, 1.5571000855431985, 1.5571000855431985, 1.5571000855431985, 1.5571000855431985, 1.5571000855431985, 1.5571000855431985, 1.5571000855431985, 1.5571000855431985, 1.5571000855431985, 1.5571000855431985, 1.5571000855431985, 1.5571000855431985, 1.5571000855431985, 1.5571000855431985, 1.5571000855431985, 1.5571000855431985, 1.5571000855431985, 1.5571000855431985, 1.5571000855431985, 1.5571000855431985, 1.5571000855431985, 1.5571000855431985, 1.5571000855431985, 1.5571000855431985, 1.5571000855431985, 1.5571000855431985, 1.5571000855431985, 1.5571000855431985, 1.5571000855431985, 1.5571000855431985, 1.5571000855431985, 1.5571000855431985, 1.5571000855431985, 1.5571000855431985, 1.5571000855431985, 1.5571000855431985, 1.5571000855431985, 1.5571000855431985, 1.5571000855431985, 1.5571000855431985, 1.5571000855431985, 1.5571000855431985, 1.5571000855431985, 1.5571000855431985, 1.5571000855431985, 1.5571000855431985, 1.5571000855431985, 1.5571000855431985, 1.5571000855431985, 1.5571000855431985, 1.5571000855431985, 1.5571000855431985, 1.5571000855431985, 1.5571000855431985, 1.5571000855431985, 1.5571000855431985, 1.5571000855431985, 1.5571000855431985, 1.5571000855431985, 1.5571000855431985, 1.5571000855431985, 1.5571000855431985, 1.5571000855431985, 1.5571000855431985, 1.5571000855431985, 1.5571000855431985, 1.5571000855431985, 1.5571000855431985, 1.5571000855431985, 1.5571000855431985, 1.5571000855431985, 1.5571000855431985, 1.5571000855431985, 1.5571000855431985, 1.5571000855431985, 1.5571000855431985, 1.5571000855431985, 1.5571000855431985, 1.5571000855431985, 1.5571000855431985, 1.5571000855431985, 1.5571000855431985]
  out "beak":dbl[](graph)=[3.5, 3.5, 3.5, 3.5, 3.5, 3.5, 3.5, 3.5, 3.5, 3.5, 3.5, 3.5, 3.5, 3.5, 3.5, 3.5, 3.5, 3.5, 3.5, 3.5, 3.5, 3.5, 3.5, 3.5, 3.5, 3.5, 3.5, 3.5, 3.5, 3.5, 3.5, 3.5, 3.5, 3.5, 3.5, 3.5, 3.5, 3.5, 3.5, 3.5, 3.5, 3.5, 3.5, 3.5, 3.5, 3.5, 3.5, 3.5, 3.5, 3.5, 3.5, 3.5, 3.5, 3.5, 3.5, 3.5, 3.5, 3.5, 3.5, 3.5, 3.5, 3.5, 3.5, 3.5, 3.5, 3.5, 3.5, 3.5, 3.5, 3.5, 3.5, 3.5, 3.5, 3.5, 3.5, 3.5, 3.5, 3.5, 3.5, 3.5, 3.5, 3.5, 3.5, 3.5, 3.5, 3.5, 3.5, 3.5, 3.5, 3.5, 3.5, 3.5, 3.5, 3.5, 3.5, 3.5, 3.5, 3.5, 3.5, 3.5, 3.5, 1.9785542665, 1.990158996, 2.025746527, 1.9810984445, 1.9476016139999999, 1.9091485525, 1.7767422469999998, 1.7064507320000002, 1.4434325045, 1.4321563620000002, 1.3193370995000002, 1.129089612, 1.3282307675, 1.4206845205, 1.5625786435, 1.4861098735000002, 0.8281851654999999, 0.767759657, 0.8309755825000003, 0.18382533399999978, 0.2123986095000001, 0.2166976945000001, 0.42721850150000007, 0.673057896, 0.8843739100000003, 1.0535822465, 1.1190077465, 0.27683675249999995, 0.7145755364999999, 0.8848588735000003, 0.4807866769999998, 0.7829142510000002, 0.902870472, 1.004963988, 1.1526721710000003, 1.4143135755, 1.3291377715000001, 1.1963446985, 0.9521470454999998, 1.340428222, 1.4614099255, 0.8258395075, 0.6571293505, 0.7935647299999999, 0.8167256964999998, 0.7832865249999998, 0.58379146, 0.5166473480000002, 0.389139793, 0.5215624435000001, 0.5215624435000001, 0.5215624435000001, 0.5215624435000001, 0.5215624435000001, 0.9591320830000001, 0.8342912619999998, 0.6803582170000002, 0.9253731409999997, 1.2560185785, 1.2140250149999998, 0.3961297199999998, 0.04530298850000003, 0.005176443999999947, 0.5129740665, 0.6392993634999997, 0.16943211950000014, 0.08139519499999981, 0.13478297699999997, 0.6184511585000001, 0.705219907, 0.711514636, 0.7737119775000001, 0.9311584625, 1.0457033965, 1.0028120024999998, 0.700202902, 0.7133278249999999, 1.1859852269999998, 0.9916243680000001, 0.0, 0.19709861149999996, 0.363616484, 0.6735513295, 1.0981670525, 1.4083660290000002, 1.3015658985000003, 1.2600938805, 1.183977879, 0.5450892475, 0.5215624435000001, 1.5143749635000001, 2.50718748, 3.00359374, 3.00359374, 3.00359374, 3.00359374, 3.00359374, 2.5402301224999997, 2.3540466635, 2.2153703985, 2.022575044, 1.9852982555, 2.0151073459999997, 1.92416308, 1.7075639455, 1.8680117295, 1.9225440045, 1.9344812095000001, 1.976313633, 2.2460896255, 2.5522391825, 2.6934785254999998, 2.1759045665, 1.814401344, 2.2218734335, 1.5788869705, 1.2318035694999998, 1.3896128435000001, 1.553914103, 1.752382891, 1.9746775964999999, 2.064387836, 2.173071152, 1.6307489134999997, 1.5921405185, 1.857376437, 1.6037078015, 1.6377744845000002, 1.736922726, 1.7398913735, 1.962444708, 2.2526244965, 2.343694801, 2.1685017479999997, 2.3411281004999998, 2.4461943379999997, 3.00359374, 3.00359374, 3.00359374, 3.00359374, 3.00359374, 2.516549266, 2.4890678855, 2.244661454, 2.2060226335, 2.317718004, 2.4244832745, 2.4338289955, 2.4761544884999998, 2.5419128735000003, 2.56745027, 2.7031545485, 2.1929178635, 2.056870515, 2.662392243, 3.381732746, 2.8013132945, 1.6889020504999999, 1.1887527749999998, 0.7874994470000001, 1.9786805815, 2.123557597, 1.4118168225, 1.2214704145000002, 1.3750645369999996, 1.5790875450000001, 1.8663403255000002, 2.148082657, 2.415657699, 2.483056975, 2.5261431895, 2.4613459955, 2.334360693, 2.2271430055000003, 2.5481955835, 3.0503971925, 1.61427595, 0.740264217, 0.6857335170000001, 1.8806652235, 2.7784632295, 3.5, 3.5, 3.5, 3.5, 3.5, 3.5, 3.5, 3.5, 3.5, 3.5, 3.5, 3.5, 3.5, 3.5, 3.5, 3.5, 3.5, 3.5, 3.5, 3.5, 3.5, 3.5, 3.5, 3.5, 3.5, 3.5, 3.5, 3.5, 3.5, 3.5, 3.5, 3.5, 3.5, 3.5, 3.5, 3.5, 3.5, 3.5, 3.5, 3.5, 3.5, 3.5, 3.5, 3.5, 3.5, 3.5, 3.5, 3.5, 3.5, 3.5, 3.5, 3.5, 3.5, 3.5, 3.5, 3.5, 3.5, 3.5, 3.5, 3.5, 3.5, 3.5, 3.5, 3.5, 3.5, 3.5, 3.5, 3.5, 3.5, 3.5, 3.5, 3.5, 3.5, 3.5, 3.5, 3.5, 3.5, 3.5, 3.5, 3.5, 3.5, 3.5, 3.5, 3.5, 3.5, 3.5, 3.5, 3.5, 3.5, 3.5, 3.5, 3.5, 3.5, 3.5, 3.5, 3.5, 3.5, 3.5, 3.5, 3.5, 3.5, 3.5, 3.5, 3.5, 3.5, 3.2493819225, 2.984604126, 3.0406277965, 2.8525943075, 2.7116642, 2.8999121445, 3.125960579, 3.233378771, 3.171767865, 2.5433149105, 2.5532895955, 2.5835558595, 1.7892340585, 1.6967883765, 2.110174206, 2.231792752, 2.360989106, 2.4772140085, 2.678504087, 2.6401450985, 2.0260851065, 2.3479729139999996, 2.465613535, 2.1762676775000003, 2.5546200260000003, 2.67225476, 2.4556348215000003, 2.727927104, 3.0518434275, 2.8637517825, 2.740663422, 2.7356930999999998, 3.027508393, 3.1991240645, 2.653731339, 2.577363061, 2.632879767, 2.6677336945, 2.6996149985, 2.640421756, 2.541002394, 2.5283850095, 2.6130134065, 2.684878196, 2.7030314325, 2.8888491625, 2.90941721, 2.862434813, 2.6994522205, 2.4823475285, 2.926836808, 3.3368261535, 3.5, 2.513780864, 1.9187025655, 1.5917112749999998, 2.163301861, 2.341835958, 2.262452759, 1.8607341339999999, 1.9022359895, 2.3398385605, 2.481996097, 2.5683760655, 2.9237967535, 2.9332865135, 2.7618196445, 2.746826187, 2.7010902765, 2.9040290895, 3.4805411795, 0.7201249475, 0.5215624435000001, 1.0891961955, 1.4869182545, 1.8705900115, 2.3746880150000003, 2.6354126365, 2.8848548574999997, 2.601234797, 2.3141729555, 1.7093608630000001, 1.594604816, 1.943860751, 1.6993908575, 1.70892127, 1.9671975155, 2.1839977284999996, 2.2318820859999997, 2.4345890695000003, 2.561069756, 2.535234044, 2.478517566, 2.2632863084999997, 2.076136104, 1.944416768, 1.846498052, 1.8784317755, 1.5767109785, 1.7433518060000002, 1.7342556279999999, 1.7147067945, 1.9598063135000001, 2.2913395784999997, 2.5684218175, 2.5187700195, 1.7055816225, 1.5970582949999999, 1.820895244, 1.0480351595, 1.1017480809999998, 1.118909694, 1.3676689565000002, 1.6877462245000001, 1.7077263979999997, 1.0179687034999998, 0.02515618350000004, 1.0179687034999998, 0.8235628555000001, 1.4777921900000002, 1.3656231225000002, 1.3254201239999999, 1.4389862130000002, 1.3738828879999998, 1.4506004729999997, 1.9846123115, 1.9023562075, 1.5872395384999998, 2.0546706845, 1.943299967, 2.5017715555, 2.0456556155, 1.853562417, 1.3890834964999996, 1.6871119685000002, 1.8532878174999998, 1.8945143455, 1.7833169795000001, 1.5785892885, 1.5007818140000002, 1.1497961405, 1.5962251795000002, 1.639252188, 1.6475762134999998, 1.698384548, 1.6472040620000001, 1.3539543255000002, 1.0874447430000003, 1.622370939, 2.0029607604999997, 2.0760186335, 1.1819242399999998, 0.9016465884999998, 0.02515618350000004, 1.0179687034999998, 1.712937464, 1.5143749635000001, 0.7201249475, 0.8382658059999999, 1.1153346295, 1.3092856805, 1.3715100699999998, 1.461975571, 1.5845231919999998, 1.516991105, 1.4487442444999998, 1.4116473875, 1.3958444115000002, 1.4250988149999997, 1.276092797, 0.7155141629999999, 0.07665919799999976, 0.09203880699999978, 0.5363435875000002, 1.1342049109999999, 1.659728049, 1.8674685435, 1.746019821, 1.7954805645, 1.844536561, 1.4100235310000002, 0.9369200260000001, 1.257586071, 0.9366959105000001, 0.8955475305, 1.413672757, 1.4542856719999997, 1.4234215135000001, 1.686860616, 1.9469646455, 1.9328354255, 1.775105738, 1.5903850059999998, 1.6444706985, 1.5098870815, 1.6296031990000002, 1.812261318, 1.7134324689999998, 1.8417018164999999, 3.5, 3.5, 3.5, 3.5, 3.5, 3.5, 3.5, 3.5, 3.5, 3.5, 3.5, 3.5, 3.5, 3.5, 3.5, 3.5, 3.5, 3.5, 3.5, 3.5, 3.5, 3.5, 3.5, 3.5, 3.5, 3.5, 3.5, 3.5, 3.5, 3.5, 3.5, 3.5, 3.5, 3.5, 3.5, 3.5, 3.5, 3.5, 3.5, 3.5, 3.5, 3.5, 3.5, 3.5, 3.5, 3.5, 3.5, 3.5, 3.5, 3.5, 3.5, 3.5, 3.5, 3.5, 3.5, 3.5, 3.5, 3.5, 3.5, 3.5, 3.5, 3.5, 3.5, 3.5, 3.5, 3.5, 3.5, 3.5, 3.5, 3.5, 3.5, 3.5, 3.5, 3.5, 3.5, 3.5, 3.5, 3.5, 3.5, 3.5, 3.5, 3.5, 3.5, 3.5, 3.5, 3.5, 3.5, 3.5, 3.5, 3.5, 3.5, 3.5, 3.5, 3.5, 3.5, 3.5, 3.5, 3.5, 3.5, 3.5, 3.5, 3.5, 3.5, 3.5, 3.5, 3.5, 3.5, 3.5, 3.5, 3.5, 3.5, 3.5, 3.5, 3.5, 3.5, 3.5, 3.5, 3.5, 3.5, 3.5, 3.5, 3.5, 3.5, 3.5, 3.5, 3.5, 3.5, 3.5, 3.5, 3.5, 3.5, 3.5, 3.5, 3.5, 3.5, 3.5, 3.5, 3.5, 3.5, 3.5, 3.5, 3.5, 3.5]
  # "play certain file"
  # "Time Period"
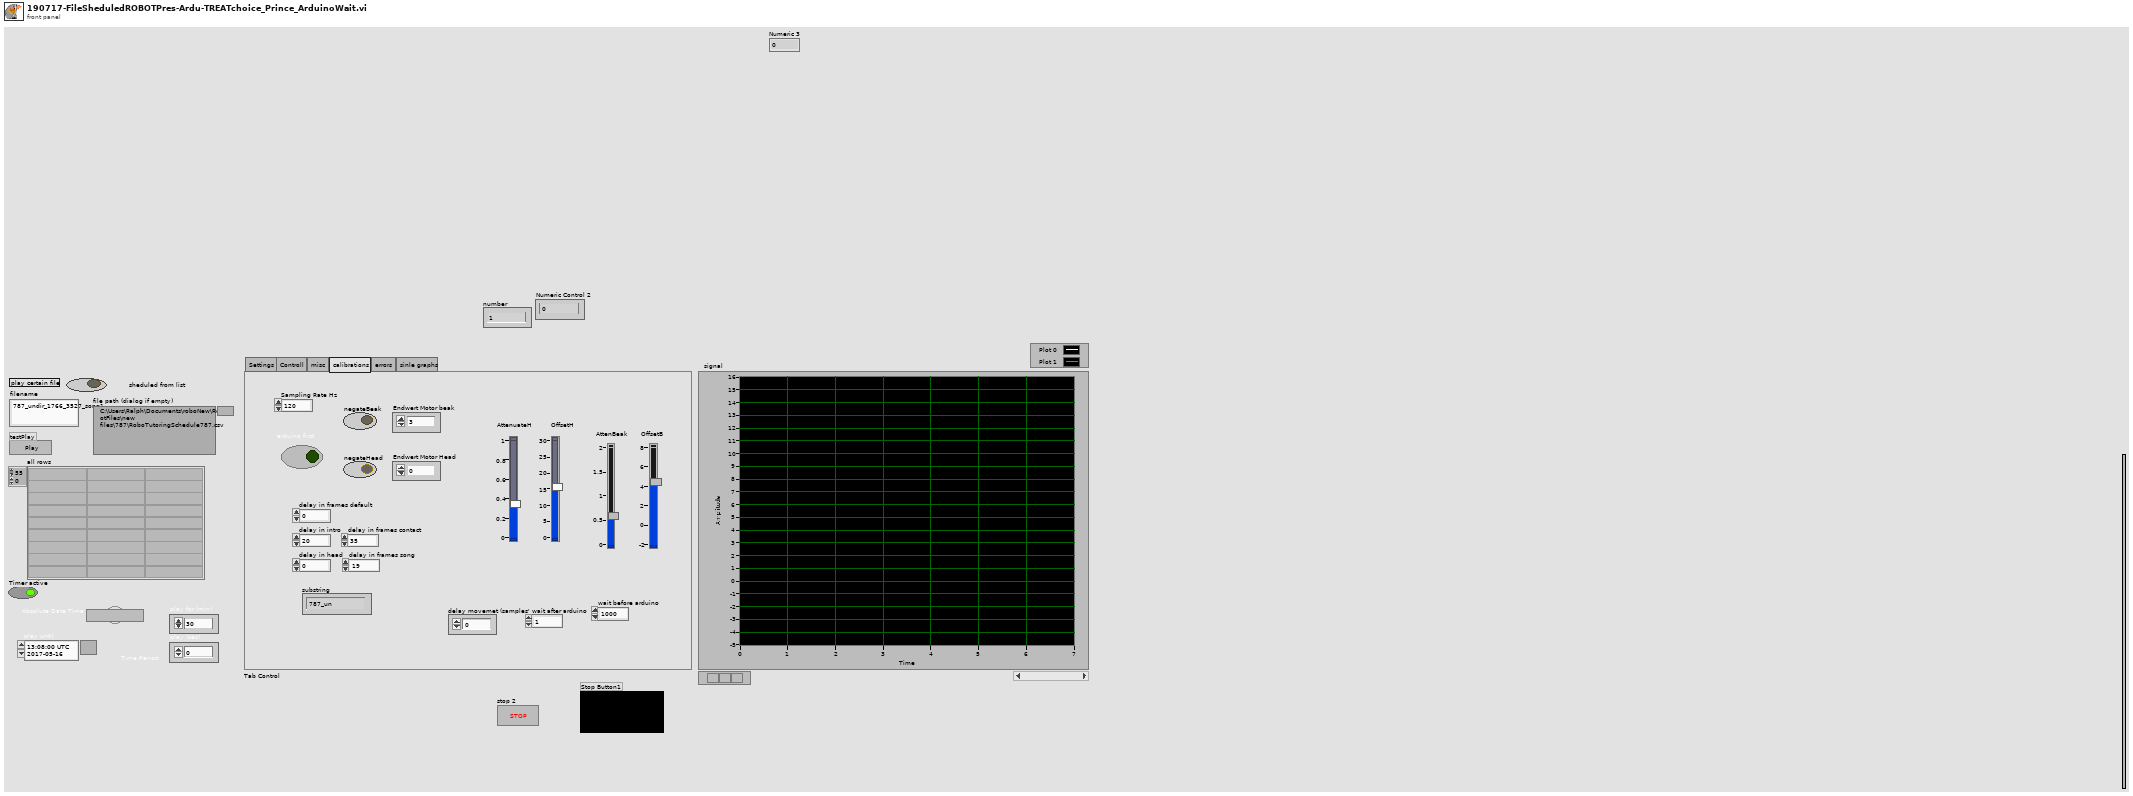
[diagram p1: front panel]
types:
  T1 = enum32{"Settings", "Controll", "misc", "calibrations", "errors", "sinle graphs"}
  T2 = enum16{"open", "replace", "create", "open or create", "replace or create", "replace or create with confirmation"}
  T3 = typedef "Sound Data Format.ctl" = cluster{"sample rate (S/s)":dbl, "number of channels":i32, "bits per sample":i32}
  T4 = typedef "Sampling Mode.ctl" = i32
  T5 = typedef "Sound Output Task ID.ctl" = u32
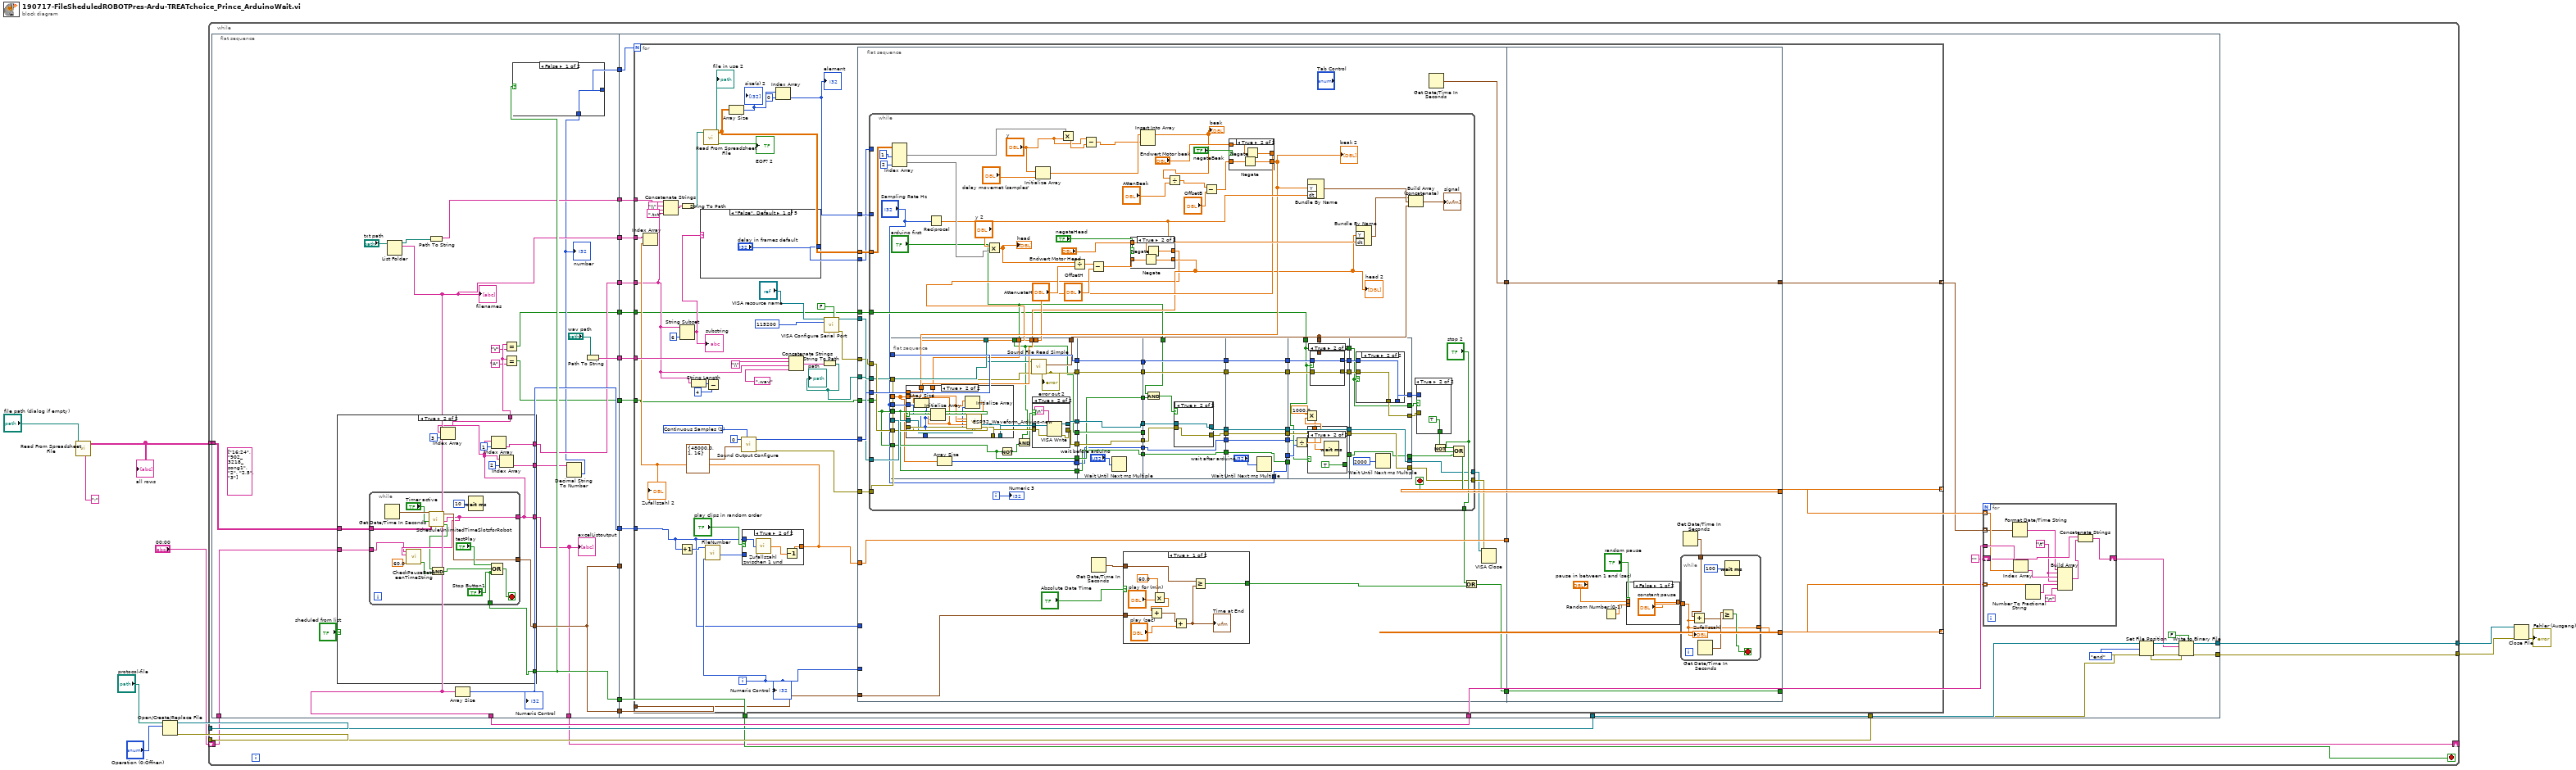
[diagram p0: block diagram]
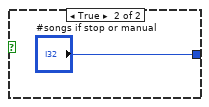
[diagram p2: hidden frame]
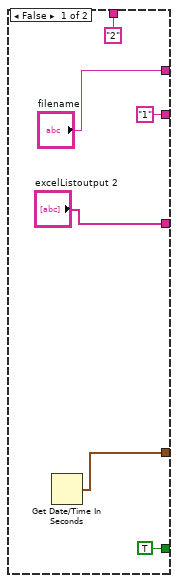
[diagram p3: hidden frame]
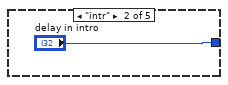
[diagram p4: hidden frame]
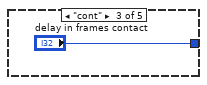
[diagram p5: hidden frame]
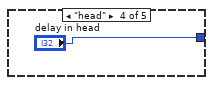
[diagram p6: hidden frame]
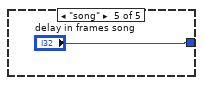
[diagram p7: hidden frame]
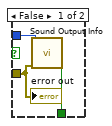
[diagram p9: hidden frame]
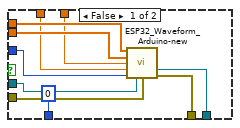
[diagram p12: hidden frame]
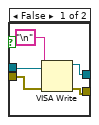
[diagram p14: hidden frame]
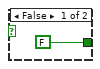
[diagram p15: hidden frame]
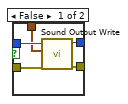
[diagram p16: hidden frame]
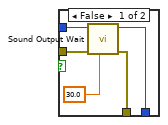
[diagram p17: hidden frame]
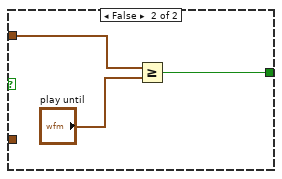
[diagram p18: hidden frame]
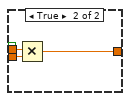
[diagram p19: hidden frame]
diagram:
  n1 = call-poly <vilib>:"Read From Spreadsheet File.vi"("delimiter (\\t)"=";" ("delimiter (\\t)"), "file path (dialog if empty)"="file path (dialog if empty)") -> ("all rows"=w4:string[][])  [unwired: 5 in, 4 out]
  "all rows" <- w4
  n2 = Open/Create/Replace File(file path (use dialog)="protocol-file", operation (0:open)="Operation (0:Öffnen)") -> (refnum out=w11:refnum<file>, error out=w10:errorcluster)  [unwired: 4 in, 1 out]
  n3 = while {
    tunnel: w11 -> [w26]
    tunnel: w10 -> [w25]
    tunnel: [w24] -> w6
    tunnel: [w23] -> w5
    tunnel: w4 -> [w18]
    shift-right: [w15] -> _
    shift-left: "00:00" -> [w14]
    stop <- w16 stop-if-true
    n4 = flat-sequence {
      tunnel: [w50] -> w31
      tunnel: [w53] -> w30
      tunnel: [w53] -> w29
      tunnel: [w51] -> w28
      tunnel: [w43] -> w27
      tunnel: [w49] -> w22
      tunnel: [w43] -> w21
      tunnel: [w45] -> w20
      tunnel: [w44] -> w19
      tunnel: w18 -> [w42]
      tunnel: [w41] -> w17
      tunnel: [w40] -> w15
      tunnel: w14 -> [w39]
      tunnel: [w33] -> w13
      tunnel: [w32] -> w12
      tunnel: w31 -> [w110]
      tunnel: w30 -> [_]
      tunnel: w29 -> [w109]
      tunnel: w28 -> [w108]
      tunnel: [w108] -> w16
      tunnel: w27 -> [w106]
      tunnel: w26 -> [w99]
      tunnel: w25 -> [w98]
      tunnel: [w96] -> w24
      tunnel: [w95] -> w23
      tunnel: w22 -> [w89]
      tunnel: w21 -> [w93]
      tunnel: w20 -> [w92]
      tunnel: w19 -> [w91]
      tunnel: w17 -> [w90]
      tunnel: w13 -> [w88]
      tunnel: w12 -> [w87]
      frame #0 {
        (unwired) string[] ["16:24", "902_3218_song1", "2", "2,5", "3"] ("excelListoutput 3")
        n5 = case shown="True" "sheduled from list" {
          tunnel: [w61 w71] -> w53
          tunnel: [TRUE ("Stop Button1") w72] -> w51
          tunnel: w42 -> [_ w70]
          tunnel: ["excelListoutput 2" w63] -> w40
          tunnel: ["filename" w68] -> w41
          tunnel: w39 -> [_ w67]
          tunnel: ["1" w65] -> w38
          tunnel: ["2" w62] -> w36
          frame False {
            n6 = Get Date/Time In Seconds() -> (seconds since 1Jan1904=w61:timestamp)
          }
          frame True {
            n7 = while {
              tunnel: ["Stop Button1"] -> w72
              tunnel: [w79] -> w71
              tunnel: w70 -> [w81]
              tunnel: [w78] -> w63
              tunnel: w67 -> [w73]
              stop <- w85 stop-if-true
              n8 = Get Date/Time In Seconds() -> (seconds since 1Jan1904=w82:timestamp)
              n9 = call "ScheduleUnlimitedTimeSlotsforRobot.vi"("excelList"=w81, "Timer active"="Timer active", "current time"=w82) -> ("activation"=w75:bool, "Array 2"=w78:string[], "current time"=w79:timestamp)  [unwired: 3 in, 1 out]
              n10 = call "CheckPauseBetweenTimeString.vi"("greater than (s)"=60.0, "laterEntry"=w78, "earlierEntry"=w73) -> ("pause ok"=w76:bool)  [unwired: 7 in, 1 out]
              n11 = And(x=w75, y=w76) -> (x .and. y?=w74:bool)
              n12 = Wait (ms)(milliseconds to wait=u32 10) -> ()  [unwired: 1 out]
              n13 = Compound Arithmetic op=OR("testPlay", w74, "Stop Button1") -> (w85:bool)
            }
            n14 = Index Array(array=w63, index=3) -> (element=w62:string)
            n15 = Index Array(array=w63, index=1) -> (element=w68:string)
            n16 = Index Array(array=w63, index=2) -> (element=w65:string)
          }
        }
        "excelListoutput" <- w40
        n17 = List Folder(path="txt path") -> (path out=w47:path, filenames=w43:string[])  [unwired: 3 in, 2 out]
        "filenames" <- w43
        n18 = Path To String(path=w47) -> (string=w45:string)
        n19 = Array Size(array=w43) -> (size(s)=w50:i32)
        "Numeric Control" <- w50
        n20 = Equal?(x=w36, y="V") -> (x = y?=w32:bool)
        n21 = Equal?(x=w36, y="A") -> (x = y?=w33:bool)
        n22 = Decimal String To Number(string=w38) -> (number=w37:i32)  [unwired: 2 in, 1 out]
        "number" <- w37
        n23 = case shown="False" w51 {
          tunnel: [w54 "#songs if stop or manual"] -> w49
          tunnel: w37 -> [w54 _]
          frame False {
          }
          frame True {
          }
        }
        n24 = Path To String(path="wav path") -> (string=w44:string)
      }
      frame #1 {
        n25 = for {
          N: w89 -> [_]
          tunnel: w110 -> [w125]
          tunnel: w109 -> [w158]
          tunnel: [w155] -> w107 mode=indexing
          tunnel: [w154] -> w105 mode=indexing
          tunnel: [w152] -> w104 mode=indexing
          tunnel: w93 -> [w141]
          tunnel: w92 -> [w138]
          tunnel: w91 -> [w131]
          tunnel: w90 -> [w113]
          tunnel: w88 -> [w112]
          tunnel: w87 -> [w111]
          i -> [w148]
          w129 = T4 1 items=["Finite Samples", "Continuous Samples"] ("sample mode")
          n26 = Concatenate Strings(w138, "\\" ("string"), w113, ".txt" ("string")) -> (w140:string)
          n27 = Increment(x=w125) -> (x+1=w149:i32)
          n28 = String To Path(string=w140) -> (path=w137:path)
          n29 = String Subset(string=w113, length (rest)=6 ("length (rest)")) -> (substring=w121:string)  [unwired: 1 in]
          "substring" <- w121
          n30 = String Length(string=w113) -> (length=w135:i32)
          n31 = case shown="\"False\", Default" w121 {
            tunnel: ["delay in frames default" "delay in intro" "delay in frames contact" "delay in head" "delay in frames song"] -> w123
            frame "False", Default {
            }
            frame "intr" {
            }
            frame "cont" {
            }
            frame "head" {
            }
            frame "song" {
            }
          }
          n32 = call-poly <vilib>:"Read From Spreadsheet File.vi"("file path (dialog if empty)"=w137) -> ("EOF?"=→"EOF? 2":bool, "all rows"=w143:dbl[][], "new file path (Not A Path if cancelled)"=→"file in use 2":path)  [unwired: 6 in, 2 out]
          n33 = call "FileNumber.vi"("LoopIteration"=w148, "NumberFiles"=w149) -> ("FileNumber"=w150:i32)  [unwired: 9 in]
          n34 = Subtract(x=w135, y=4) -> ()  [unwired: 1 out]
          n35 = Array Size(array=w143) -> (size(s)=w145:i32[])
          "size(s) 2" <- w145
          n36 = call <vilib>:"Sound Output Configure.vi"("sample mode"=w129, "sound format"=T3 {"sample rate (S/s)"=48000.0, "number of channels"=1, "bits per sample"=16}, "device ID"=u32 0) -> ("error out"=w126:errorcluster, "task ID"=w127:T5)  [unwired: 7 in]
          n37 = case shown="True" "play clips in random order" {
            tunnel: w125 -> [_ w167]
            tunnel: [w164 w165] -> w124
            tunnel: w150 -> [w164 _]
            frame False {
            }
            frame True {
              n38 = call "Zufallszahl zwischen 1 und.vi"("Zufallszahl \nzwischen 1 und"=w167) -> ("Zufallszahl"=w166:dbl)
              n39 = Decrement(x=w166) -> (x-1=w165:dbl)
            }
          }
          "Zufallszahl 2" <- w124
          n40 = Index Array(array=w141, index=w124) -> ()  [unwired: 1 out]
          n41 = Index Array(array=w145, index=0) -> (element=w142:i32)
          "element" <- w142
          n42 = Concatenate Strings(w131, "\\" ("string"), w113, ".wav" ("string")) -> (w136:string)
          n43 = String To Path(string=w136) -> (path=w115:path)
          "path" <- w115
          n44 = call-poly "VISA Configure Serial Port"("VISA resource name"="VISA resource name", "Enable Termination\nChar (T)"=FALSE ("Enable Termination\nChar (T)"), "baud rate (9600)"=u32 115200) -> ("VISA resource name out"=w118:refnum<visa-resource-name>, "error out"=w117:errorcluster)  [unwired: 11 in]
          n45 = flat-sequence {
            tunnel: w158 -> [w186]
            tunnel: [w183] -> w157
            tunnel: w125 -> [_]
            tunnel: [w181] -> w156
            tunnel: [w182] -> w153
            tunnel: w148 -> [_]
            tunnel: w124 -> [w181]
            tunnel: w143 -> [w180]
            tunnel: w142 -> [w179]
            tunnel: w127 -> [w178]
            tunnel: w115 -> [w177]
            tunnel: w126 -> [w176]
            tunnel: w123 -> [w174]
            tunnel: w118 -> [w173]
            tunnel: w117 -> [w172]
            tunnel: w112 -> [w169]
            tunnel: w111 -> [w168]
            tunnel: [w438] -> _
            tunnel: w157 -> [w438]
            tunnel: w156 -> [w436]
            tunnel: [w436] -> w155
            tunnel: [w435] -> w154
            tunnel: w153 -> [w434]
            tunnel: [w434] -> w152
            frame #0 {
              n46 = while {
                tunnel: w180 -> [w268]
                tunnel: w179 -> [_]
                tunnel: w178 -> [w274]
                tunnel: w177 -> [w237]
                tunnel: w176 -> [w238]
                tunnel: ["stop 2"] -> w175
                tunnel: w174 -> [_]
                tunnel: w173 -> [w260]
                tunnel: w172 -> [w259]
                tunnel: [w258] -> w171
                tunnel: [w227] -> w170
                tunnel: w169 -> [w205]
                tunnel: w168 -> [w202]
                i -> [w275]
                stop <- w271 stop-if-true
                n47 = flat-sequence {
                  tunnel: [w314] -> w243
                  tunnel: w274 -> [w314]
                  tunnel: w218 -> [w313]
                  tunnel: w225 -> [w294]
                  tunnel: w217 -> [w312]
                  tunnel: w224 -> [w311]
                  tunnel: "Sampling Rate Hz" -> [w310]
                  tunnel: w260 -> [w309]
                  tunnel: w259 -> [w300]
                  tunnel: [w299] -> w242
                  tunnel: [w303] -> w240
                  tunnel: "arduino first" -> [w299]
                  tunnel: w238 -> [w308]
                  tunnel: w237 -> [w307]
                  tunnel: [w306] -> w236
                  tunnel: [w305] -> w214
                  tunnel: [w301] -> w229
                  tunnel: w205 -> [w295]
                  tunnel: w205 -> [w296]
                  tunnel: [w296] -> w203
                  tunnel: [w295] -> w196
                  tunnel: [w293] -> w188
                  tunnel: w243 -> [w346]
                  tunnel: w242 -> [w351]
                  tunnel: [w351] -> w241
                  tunnel: w240 -> [w350]
                  tunnel: [w350] -> w239
                  tunnel: w236 -> [w347]
                  tunnel: [w348] -> w230
                  tunnel: w229 -> [w348]
                  tunnel: [w346] -> w216
                  tunnel: [w347] -> w213
                  tunnel: [w345] -> w204
                  tunnel: w203 -> [w345]
                  tunnel: [w344] -> w197
                  tunnel: w196 -> [w344]
                  tunnel: [w343] -> w189
                  tunnel: w188 -> [w343]
                  tunnel: w241 -> [_]
                  tunnel: w239 -> [w357]
                  tunnel: [w358] -> w253
                  tunnel: [w361] -> w251
                  tunnel: [w362] -> w249
                  tunnel: [w359] -> w231
                  tunnel: w230 -> [w360]
                  tunnel: w216 -> [w361]
                  tunnel: "arduino first" -> [w355]
                  tunnel: w213 -> [w362]
                  tunnel: w204 -> [w356]
                  tunnel: [w353] -> w198
                  tunnel: w197 -> [w353]
                  tunnel: [w352] -> w190
                  tunnel: w189 -> [w352]
                  tunnel: w253 -> [w377]
                  tunnel: [w377] -> w252
                  tunnel: w251 -> [w376]
                  tunnel: [w376] -> w250
                  tunnel: w249 -> [w375]
                  tunnel: [w375] -> w248
                  tunnel: [w373] -> w232
                  tunnel: w231 -> [w373]
                  tunnel: [w372] -> w201
                  tunnel: "Sampling Rate Hz" -> [w372]
                  tunnel: [w371] -> w199
                  tunnel: w198 -> [w371]
                  tunnel: [w370] -> w191
                  tunnel: w190 -> [w370]
                  tunnel: w252 -> [w390]
                  tunnel: w250 -> [w389]
                  tunnel: w248 -> [w387]
                  tunnel: [w386] -> w255
                  tunnel: [w385] -> w254
                  tunnel: w232 -> [w391]
                  tunnel: [w391] -> w228
                  tunnel: [w390] -> w226
                  tunnel: w214 -> [w388]
                  tunnel: w202 -> [w379]
                  tunnel: w201 -> [w384]
                  tunnel: w199 -> [_]
                  tunnel: [w383] -> w195
                  tunnel: [w379] -> w193
                  tunnel: w191 -> [w378]
                  tunnel: [w409] -> w256
                  tunnel: [w407] -> w257
                  tunnel: [w404] -> w258
                  tunnel: w255 -> [w408]
                  tunnel: w254 -> [w410]
                  tunnel: [w405] -> w227
                  tunnel: w228 -> [w405]
                  tunnel: w226 -> [w404]
                  tunnel: w195 -> [w403]
                  tunnel: [w403] -> w194
                  tunnel: w193 -> [w402]
                  tunnel: [w402] -> w192
                  frame #0 {
                    n48 = case shown="True" w295 {
                      tunnel: w313 -> [w324 w331]
                      tunnel: w294 -> [w323 _]
                      tunnel: w312 -> [w322 w329]
                      tunnel: w311 -> [w321 w330]
                      tunnel: w310 -> [w320 w328]
                      tunnel: w309 -> [w319 w334]
                      tunnel: w300 -> [w318 w335]
                      tunnel: [w317 w333] -> w304
                      tunnel: [w316 w332] -> w302
                      tunnel: [0 w325] -> _
                      frame False {
                        n49 = call "ESP32_Waveform_Arduino-new.vi"("headMove"=w324, "beakMove"=w323, "Endwert Motor1"=w322, "Endwert Motor2"=w321, "Sampling Rate Hz"=w320, "VISA resource name in"=w319, "error in"=w318) -> ("VISA resource name out"=w316:refnum<visa-resource-name>, "error out"=w317:errorcluster)  [unwired: 7 in]
                      }
                      frame True {
                        n50 = Array Size(array=w331) -> (size(s)=w325:i32)
                        n51 = Initialize Array(w330, w325) -> (w327:dbl[])
                        n52 = Initialize Array(w329, w325) -> (w326:dbl[])
                        n53 = call "ESP32_Waveform_Arduino-new.vi"("headMove"=w326, "beakMove"=w327, "Endwert Motor1"=w329, "Endwert Motor2"=w330, "Sampling Rate Hz"=w328, "VISA resource name in"=w334, "error in"=w335) -> ("VISA resource name out"=w332:refnum<visa-resource-name>, "error out"=w333:errorcluster)  [unwired: 7 in]
                      }
                    }
                    n54 = Array Size(array=w294) -> (size(s)=w293:i32)
                    n55 = Not(x=w296) -> (.not. x?=w297:bool)
                    n56 = And(x=w299, y=w297) -> (x .and. y?=w298:bool)
                    n57 = call <vilib>:"Sound File Read Simple.vi"("error in (no error)"=w308, "path"=w307) -> ("error out"=w306:errorcluster, "data"=w305:waveform(dbl)[])  [unwired: 6 in, 2 out]
                    "error out 2" <- w306
                    n58 = case shown="True" w298 {
                      tunnel: w304 -> [w336 w341]
                      tunnel: w302 -> [w337 w340]
                      tunnel: [w337 w339] -> w301
                      tunnel: [w336 w338] -> w303
                      frame False {
                      }
                      frame True {
                        n59 = VISA Write(VISA resource name=w340, write buffer="\n" ("Schreibpuffer"), error in (no error)=w341) -> (VISA resource name out=w339:refnum<visa-resource-name>, error out=w338:errorcluster)  [unwired: 1 out]
                      }
                    }
                  }
                  frame #1 {
                    n60 = Wait Until Next ms Multiple(millisecond multiple="wait before arduino") -> ()  [unwired: 1 out]
                  }
                  frame #2 {
                    n61 = And(x=w355, y=w356) -> (x .and. y?=w354:bool)
                    n62 = case shown="True" w354 {
                      tunnel: w357 -> [w366 w368]
                      tunnel: w360 -> [w365 w369]
                      tunnel: [w364 w369] -> w359
                      tunnel: [w363 w368] -> w358
                      frame False {
                        n63 = VISA Write(VISA resource name=w365, write buffer="\n" ("Schreibpuffer"), error in (no error)=w366) -> (VISA resource name out=w364:refnum<visa-resource-name>, error out=w363:errorcluster)  [unwired: 1 out]
                      }
                      frame True {
                      }
                    }
                  }
                  frame #3 {
                    n64 = Wait Until Next ms Multiple(millisecond multiple="wait after arduino") -> ()  [unwired: 1 out]
                  }
                  frame #4 {
                    n65 = Divide(x=w378, y=w384) -> (x/y=w381:dbl)
                    n66 = Multiply(x=1000.0, y=w381) -> (x*y=w380:dbl)
                    n67 = case shown="True" w379 {
                      tunnel: [FALSE TRUE] -> w383
                      tunnel: w380 -> [_ w393]
                      frame False {
                      }
                      frame True {
                        n68 = Wait (ms)(milliseconds to wait=w393) -> ()  [unwired: 1 out]
                      }
                    }
                    n69 = case shown="True" w379 {
                      tunnel: w389 -> [w399 w400]
                      tunnel: w388 -> [w398 _]
                      tunnel: w387 -> [w397 w401]
                      tunnel: [w396 w400] -> w386
                      tunnel: [w395 w401] -> w385
                      frame False {
                        n70 = call-poly <vilib>:"Sound Output Write.vi"("error in (no error)"=w397, "data"=w398, "task ID"=w399) -> ("error out"=w395:errorcluster, "task ID out"=w396:T5)  [unwired: 7 in]
                      }
                      frame True {
                      }
                    }
                  }
                  frame #5 {
                    n71 = case shown="True" w402 {
                      tunnel: w410 -> [w415 w416]
                      tunnel: [w414 w416] -> w409
                      tunnel: w408 -> [w413 w417]
                      tunnel: [w412 w417] -> w407
                      frame False {
                        n72 = call <vilib>:"Sound Output Wait.vi"("timeout (sec)"=30.0, "error in (no error)"=w415, "task ID"=w413) -> ("error out"=w414:errorcluster, "task ID out"=w412:T5)  [unwired: 7 in]
                      }
                      frame True {
                      }
                    }
                    n73 = Wait Until Next ms Multiple(millisecond multiple=u32 2000) -> ()  [unwired: 1 out]
                  }
                }
                n74 = Index Array(array=w268, index (col) #1=1 ("disabled index (col)"), index (col) #2=2 ("disabled index (col)")) -> (element #1=w211:dbl[], element #2=w246:dbl[])  [unwired: 2 in]
                n75 = Reciprocal(x="Sampling Rate Hz") -> (1/x=w234:dbl)
                n76 = Multiply(x="y 2", y=w246) -> (x*y=w245:dbl[])
                "head" <- w245
                n77 = Initialize Array("y", "delay movemet (samples'") -> (w235:dbl[])
                n78 = Multiply(x=w211, y="y") -> (x*y=w244:dbl[])
                n79 = Divide(x=w245, y="AttenuateH") -> (x/y=w262:dbl[])
                n80 = Subtract(x="y", y=w244) -> (x-y=w210:dbl[])
                n81 = Subtract(x=w262, y="OffsetH") -> (x-y=w219:dbl[])
                n82 = case shown="True" "negateHead" {
                  tunnel: w219 -> [w281 w286]
                  tunnel: [w281 w285] -> w218
                  tunnel: [w282 w283] -> w217
                  tunnel: "Endwert Motor Head" -> [w282 w284]
                  frame False {
                  }
                  frame True {
                    n83 = Negate(x=w286) -> (-x=w285:dbl[])
                    n84 = Negate(x=w284) -> (-x=w283:dbl)
                  }
                }
                "head 2" <- w218
                n85 = Insert Into Array(array=w235, new element=w210) -> (w209:dbl[])  [unwired: 1 in]
                "beak" <- w209
                n86 = Divide(x=w209, y="AttenBeak") -> (x/y=w208:dbl[])
                n87 = Subtract(x=w208, y="OffsetB") -> (x-y=w207:dbl[])
                n88 = case shown="True" "negateBeak" {
                  tunnel: w207 -> [w287 w292]
                  tunnel: [w287 w291] -> w225
                  tunnel: [w288 w289] -> w224
                  tunnel: "Endwert Motor beak" -> [w288 w290]
                  frame False {
                  }
                  frame True {
                    n89 = Negate(x=w292) -> (-x=w291:dbl[])
                    n90 = Negate(x=w290) -> (-x=w289:dbl)
                  }
                }
                "beak 2" <- w225
                n91 = Bundle By Name("Y"=w225, "dt"=w234) -> (w269:waveform(dbl))  [unwired: 1 in]
                n92 = Bundle By Name("Y"=w218, "dt"=w234) -> (w233:waveform(dbl))  [unwired: 1 in]
                n93 = Build Array (concatenate)(w233, w269, w214) -> (→"signal":waveform(dbl)[])
                n94 = case shown="True" w192 {
                  tunnel: [w279 TRUE] -> w273
                  tunnel: w257 -> [w278 _]
                  tunnel: w256 -> [w277 _]
                  frame False {
                    n95 = call <vilib>:"Sound Output Info.vi"("error in (no error)"=w277, "task ID"=w278) -> ("is playing?"=w279:bool)  [unwired: 6 in, 3 out]
                    "error out" <- w277
                  }
                  frame True {
                  }
                }
                n96 = Not(x=w273) -> (.not. x?=w272:bool)
                n97 = Compound Arithmetic op=OR("stop 2", w272, w194) -> (w271:bool)
                "Numeric 3" <- w275
              }
              n98 = Get Date/Time In Seconds() -> (seconds since 1Jan1904=w187:timestamp)
              n99 = case shown="True" "Absolute Date Time" {
                tunnel: w187 -> [w425 w429]
                tunnel: w186 -> [w426 _]
                tunnel: [w424 w427] -> w184
                frame True {
                  n100 = Multiply(x=60.0, y="play for (min)") -> (x*y=w421:dbl)
                  n101 = Add(x=w421, y=w426) -> (x+y=w420:timestamp)
                  n102 = Add(x=w420, y="play (sec)") -> (x+y=w418:timestamp)
                  "Time at End" <- w418
                  n103 = Greater Or Equal?(x=w425, y=w418) -> (x >= y?=w424:bool)
                }
                frame False {
                  n104 = Greater Or Equal?(x=w429, y="play until") -> (x >= y?=w427:bool)
                }
              }
              n105 = Get Date/Time In Seconds() -> (seconds since 1Jan1904=w182:timestamp)
              n106 = Or(x=w175, y=w184) -> (x .or. y?=w183:bool)
              n107 = VISA Close(VISA resource name=w170, error in (no error)=w171) -> ()  [unwired: 1 out]
            }
            frame #1 {
              n108 = Random Number (0-1)() -> (number: 0 to 1=w433:dbl)
              n109 = case shown="False" "random pause" {
                tunnel: w433 -> [_ w442]
                tunnel: "pause in between 1 and (sec)" -> [_ w441]
                tunnel: ["constant pause" w440] -> w431
                frame False {
                }
                frame True {
                  n110 = Multiply(x=w441, y=w442) -> (x*y=w440:dbl)
                }
              }
              n111 = Get Date/Time In Seconds() -> (seconds since 1Jan1904=w437:timestamp)
              n112 = while {
                tunnel: w437 -> [w448]
                tunnel: w431 -> [w443]
                tunnel: [w443] -> w435
                stop <- w445 stop-if-true
                n113 = Add(x=w448, y=w443) -> (x+y=w446:timestamp)
                n114 = Get Date/Time In Seconds() -> (seconds since 1Jan1904=w447:timestamp)
                n115 = Greater Or Equal?(x=w447, y=w446) -> (x >= y?=w445:bool)
                n116 = Wait (ms)(milliseconds to wait=u32 100) -> ()  [unwired: 1 out]
                "Zufallszahl" <- w443
              }
            }
          }
          "Numeric Control 2" <- w148
        }
        n117 = for {
          tunnel: w107 -> [w459] mode=indexing
          tunnel: w106 -> [w460]
          shift-right: [w453] -> w97
          shift-left: "" -> [w454]
          tunnel: w105 -> [w458] mode=indexing
          tunnel: w104 -> [w457] mode=indexing
          w451 = "\t"
          n118 = Format Date/Time String(seconds (now)=w457) -> (date/time string=w452:string)  [unwired: 2 in]
          n119 = Index Array(array=w460, index=w459) -> (element=w456:string)
          n120 = Number To Fractional String(number=w458) -> (F-format string=w449:string)  [unwired: 3 in]
          n121 = Build Array(w452, w451, w456, w451, w449, "\n") -> (w455:string[])
          n122 = Concatenate Strings(w454, w455) -> (w453:string)
        }
        n123 = Set File Position(refnum=w99, from (0:start)=enum16{"start", "end", "current"}."end" ("Pos.-Modus (0:2)"), error in=w98) -> (refnum out=w102:refnum<file>, error out=w101:errorcluster)  [unwired: 1 in]
        n124 = Write to Binary File(file (use dialog)=w102, data=w97, error in=w101, 5:FALSE ("prepend array or string size? (T)")) -> (refnum out=w96:refnum<file>, error out=w95:errorcluster)  [unwired: 2 in, 1 out]
      }
    }
  }
  n125 = Close File(refnum=w6, error in=w5) -> (error out=→"Fehler (Ausgang)":errorcluster)  [unwired: 1 out]
